vi "Text control 2 v3.0.vi"() -> ()   [LabVIEW 2016]
panel:
  in  "Auto Reset":bool
  in  "Reset":bool
  out "Id min vs time":cluster{"Y data in":dbl[], "X data in":dbl[]}[](graph)
  in  "Start Time":dbl caption="Set Start Time (s)"
  out "Total lines":i32
  out "Line running":i32
  in  "byte count":u32=64
  in  "Serial Settings:Serial End Mode for Reads":u16(ring)=2 items=["None", "LastBit", "TermChar"]
  in  "Timeout (ms)":u32=10000
  in  "Enable Termination\nChar (T)":bool=TRUE
  in  "Termination char\n(0xA = '\\n' = LF)\n(0xD = '\\r' = CR)":u8=13 format="%.0x"
  in  "flow control":u16(ring) items=["None"=0, "XON/XOFF"=1, "RTS/CTS"=2, "DTR/DSR"=4]
  in  "stop bits":u16(ring)=10 items=["1.0"=10, "1.5"=15, "2.0"=20]
  in  "parity":u16(ring) items=["None", "Odd", "Even", "Mark", "Space"]
  in  "data bits":u16=8 min=5 max=8 step=1
  in  "VISA resource name":refnum<visa-resource-name>="COM6"
  in  "baud rate":u32=9600
  out "Serial port output":string
  out "error out":errorcluster
  in  "Units":u16(ring) items=["Seconds", "Minutes", "Hours"]
  out "Elapsed Time":dbl caption="Elapsed Time (s)"
  out "Id max vs time":cluster{"Y data in":dbl[], "X data in":dbl[]}[](graph)
  out "Ig":dbl format="%.2e"
  out "Id":dbl format="%.2e"
  out "Is":dbl format="%.2e"
  out "I vs Vg":cluster{"Y data in":dbl[], "X data in":dbl[]}[](graph)
  in  "Panel Controls 2":T1={"Emergency Stop"=refnum, "TransGraph Max"=1e-05, "Text/Graph (text=false)"=TRUE, "TransGraph Min"=1e-11} {"TransGraph Min" format="%.2e"; "TransGraph Max" format="%.2e"}
  out "Command running:":string="#output s 0 0 0 -0.008 0.008 0.002"
  in  "Standby":T2
  in  "Full Reset":bool
  in  "SMU4":cluster{"on/off":bool, "Voltage":dbl} {"Voltage" min=-100.0 max=100.0 format="%.2f"}
  in  "Source/Drain Range":u8(slide)=6 max=11 scale=0.0..11.0
  in  "Source/Drain\nRange mode":u16(ring) items=["Auto", "Limited", "Fixed"]
  in  "Gate Range":u8(slide)=6 max=11 scale=0.0..11.0
  in  "Gate Range\nmode":u16(ring) items=["Auto", "Limited", "Fixed"]
  in  "Gate":T3={"Gate Start"=0.0, "Gate Stop"=2.0, "Gate Step (linear only)"=1.0, "Gate Compliance"=0.0001, "Gate PComp"=0.0, "Range mode"=0, "Range"=6} {"Range" max=11 scale=0.0..11.0; "Range mode" items=["Auto", "Limited", "Fixed"]; "Gate PComp" format="%^.2e"; "Gate Compliance" format="%^.2e"; "Gate Step (linear only)" format="%^.4e"; "Gate Stop" format="%^.4e"; "Gate Start" format="%^.4e"}
  in  "Drain 2":T4={"Drain Start"=0.0, "Drain Stop"=2.0, "Drain Compliance"=0.0001, "Drain Step"=1.0, "Drain PComp"=0.0, "Range mode"=0, "Range"=6} {"Range" max=11 scale=0.0..11.0; "Range mode" items=["Auto", "Limited", "Fixed"]; "Drain PComp" format="%^.2e"; "Drain Step" format="%^.4e"; "Drain Compliance" format="%^.2e"; "Drain Stop" format="%^.4e"; "Drain Start" format="%^.4e"}
  in  "Timings 2":T5={"integration time"=0, "Short/Long integration time"=0.00064, "hold time (sec)"=0.0, "delay time (sec)"=0.0, "Step Time (0 disables)"=0.0, "sweep method"=0, "Pulse period"=0.005, "Base voltage"=0.0, "Pulse width"=0.0005} {"Pulse width" min=0.0005 max=0.1 step=0.0001 format="%.4f"; "Base voltage" format="%^.4e"; "Pulse period" min=0.005 max=1.0 step=0.0001 format="%.4f"; "sweep method" items=["Continuous", "Pulsed"]; "Step Time (0 disables)" format="%.2f"; "delay time (sec)" format="%.4f"; "hold time (sec)" format="%.4f"; "Short/Long integration time" format="%^.0e"; "integration time" scale=0.0..2.0}
  in  "Panel Controls":T6={"Emergency Stop"=refnum, "TransGraph Max"=1e-05, "Text/Graph (text=false)"=TRUE} {"TransGraph Max" format="%.2e"}
  in  "Interrupt run":bool
  in  "Drain: Compliance":dbl=0.001 format="%.8f"
  in  "Gate: Compliance":dbl=0.001 format="%.8f"
  out "Path":path=path "C:/users/rlp38/09Apr2009LTtesting/test2.txt"
  in  "hold time /s":dbl format="%.2f"
  in  "delay time /s":dbl format="%.2f"
  in  "integration time":u32(slide) max=2 step=1 scale=0.0..2.0
  in  "Integration time (short)":dbl=0.0019 min=8e-05 max=0.0019 step=8e-05 format="%^.0e"
  in  "Integration time (long)":dbl=0.32 min=0.04 max=2.0 step=0.02 format="%.2f"
  in  "Step delay /s":dbl format="%.2f"
  in  "Program":string="#pulsedstressV d 0.03 20 0 0.5 0.0827 5\n#\n#itime s\n#gaterangemode l\n#drainrangemode l\n#pulsed on 0.05 0 0.02\n#transfer d 1 -1 -0.1 -1 -1 0\n#wait-min 1\n#transfer d 1 -1 -0.1 -1 -1 0\n#output d 0 -1 -0.5 0 -1 -0.1\n#transfer d -10 40 1 5 40 35\n#transfer d -10 40 1 5 40 35\n#output d 0 40 20 0 40 1\n#\n#\n#sample 1 0.008 221 6 0.003\n#samplei 400e-6 200 6 0.002 0.1\n#vsu2pulse -10 4\n#\n#stressV 0.016 0.03 2e-4 0.1e-3 11\n#stressI 220e-7 0.08 15\n#transfer s -1 1 0.5 -0.005 0.005 0.005\n#output s 0 0 0 -0.008 0.008 0.002\n"
  # "Serial port settings"
  # "Time"
  # "100 samples is approx 13s with medium integration"
  # "Syntax:\nitime [s|m|l]\ngaterangemode [a|l|f]\ndrainrangemode [a|l|f]\npulsed [on|off] PulsePeriod(sec) PulseBaseVoltage PulseONWidth(sec)\nstandby [on l off]\nwait NumMilliseconds\nwait-min NumMinutes\n# texthere = comment\ntransfer [s|d] VgStart VgStop VgStep VdStart VdStop VdStep\noutput [s|d] VgStart VgStop VgStep VdStart VdStop VdStep\nsample Vg Vd NumSamples Time(s) SampleInterval(s)\nsamplei Idg NumSamples Time(s) SampleInterval(s) VDGcompliance\n# if in doubt use SampleInterval(s) = 0.004\nstressV VG VD IGcompliance IDcompliance Duration(sec)\nstressI IDG VDGcompliance Duration(sec)\nvsu2pulse Bias Duration(s)\npulsedstressV [s|d] VEstop VgON VgOFF Period(s) PulseONwidth(s) Vd\nsample-fpp Vg Vd NumSamples Time\nresample-fpp Vg Vd\ntransfer-fpp [s|d] VgStart VgStop VgStep VdStart VdStop VdStep\noutput-fpp [s|d] VgStart VgStop VgStep VdStart VdStop VdStep\nserial SerialPortCommand"
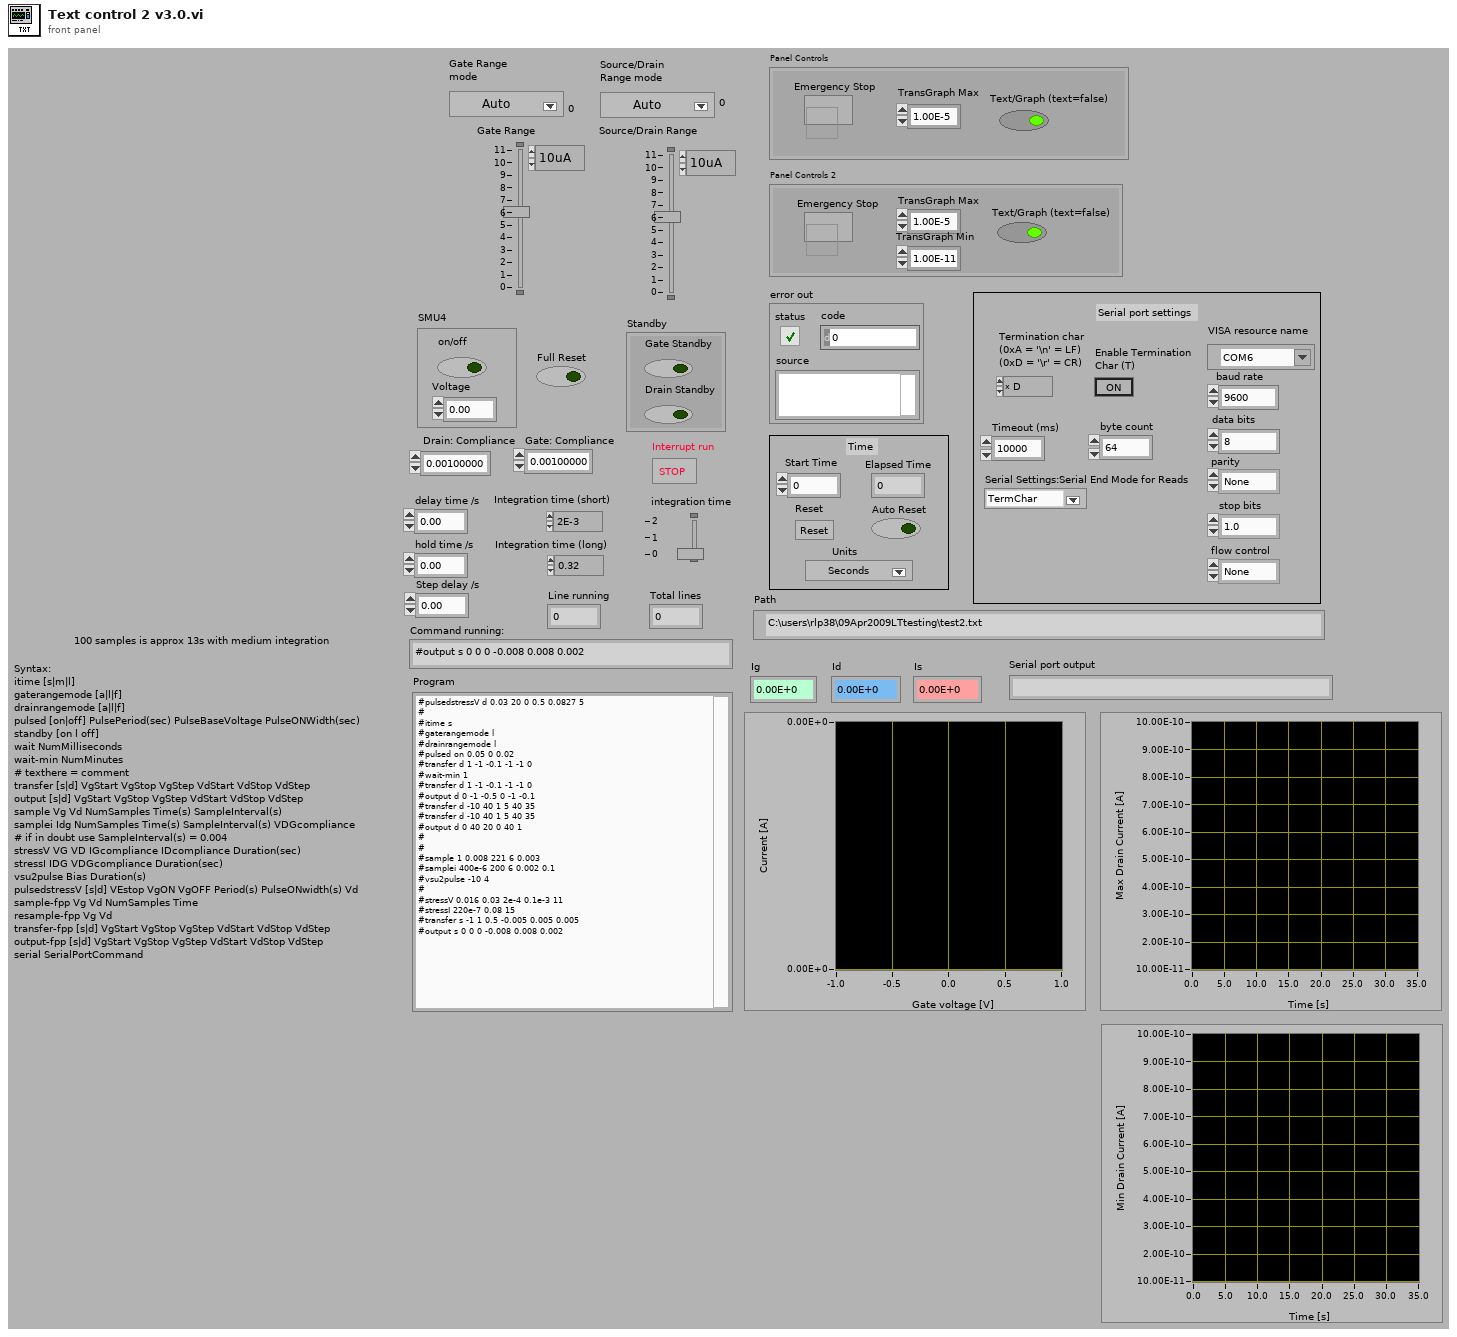
[diagram p1: front panel]
types:
  T1 = cluster{"Emergency Stop":refnum<vi>, "TransGraph Max":dbl, "Text/Graph (text=false)":bool, "TransGraph Min":dbl}
  T2 = cluster{"Gate Standby":bool, "Drain Standby":bool}
  T3 = cluster{"Gate Start":dbl, "Gate Stop":dbl, "Gate Step (linear only)":dbl, "Gate Compliance":dbl, "Gate PComp":dbl, "Range mode":u16, "Range":u8}
  T4 = cluster{"Drain Start":dbl, "Drain Stop":dbl, "Drain Compliance":dbl, "Drain Step":dbl, "Drain PComp":dbl, "Range mode":u16, "Range":u8}
  T5 = cluster{"integration time":u32, "Short/Long integration time":dbl, "hold time (sec)":dbl, "delay time (sec)":dbl, "Step Time (0 disables)":dbl, "sweep method":u16, "Pulse period":dbl, "Base voltage":dbl, "Pulse width":dbl}
  T6 = cluster{"Emergency Stop":refnum<vi>, "TransGraph Max":dbl, "Text/Graph (text=false)":bool}
  T7 = enum16{"open", "replace", "create", "open or create", "replace or create", "replace or create with confirmation"}
  T8 = cluster{"V2 Start":dbl, "V2 Step":dbl, "Number of points":i32}
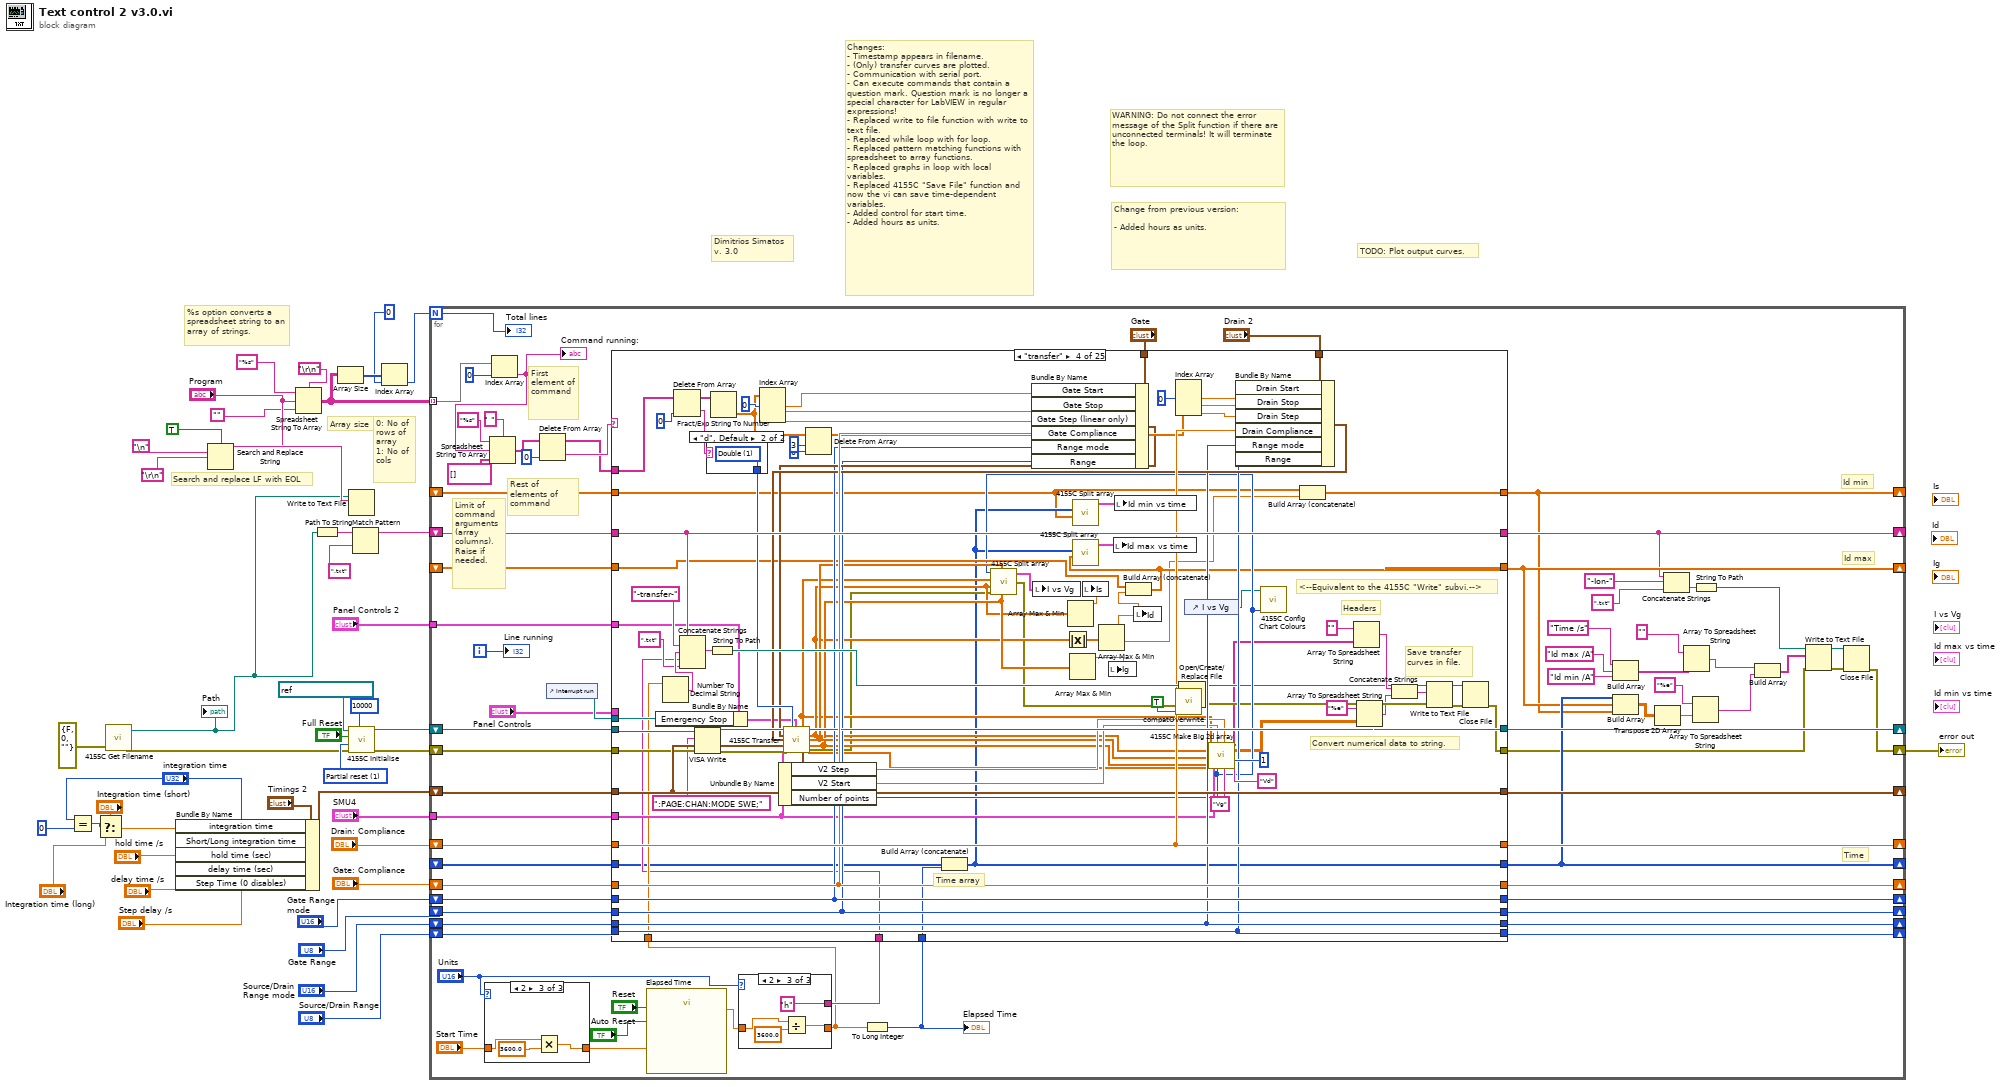
[diagram p0: block diagram]
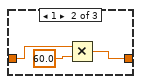
[diagram p3: hidden frame]
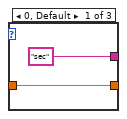
[diagram p4: hidden frame]
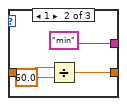
[diagram p5: hidden frame]
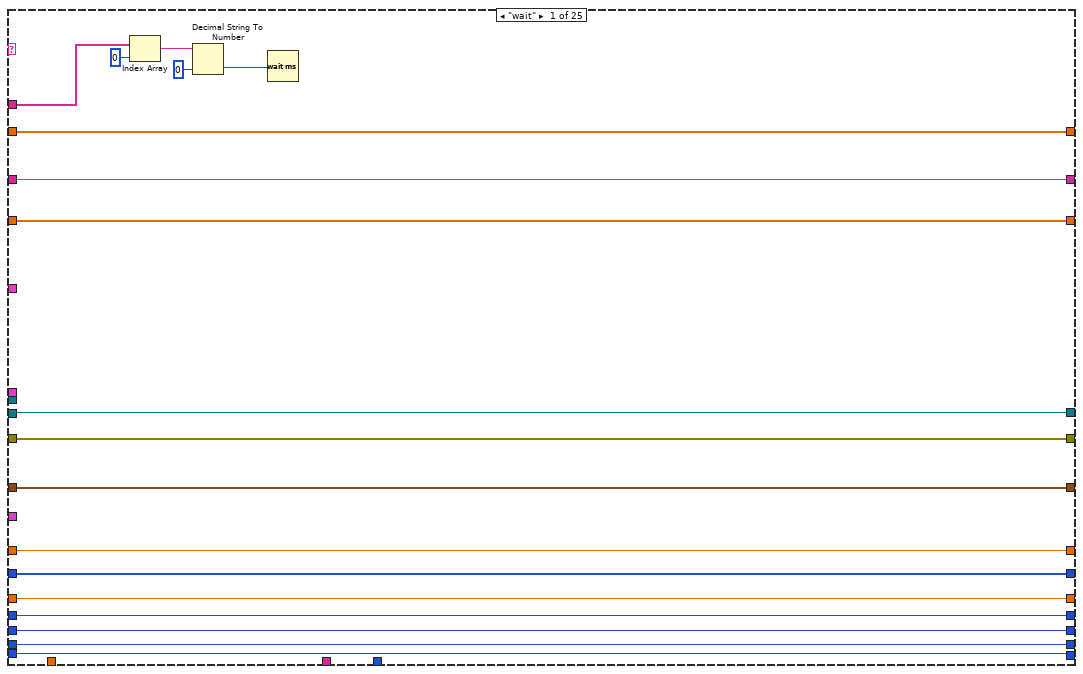
[diagram p6: hidden frame]
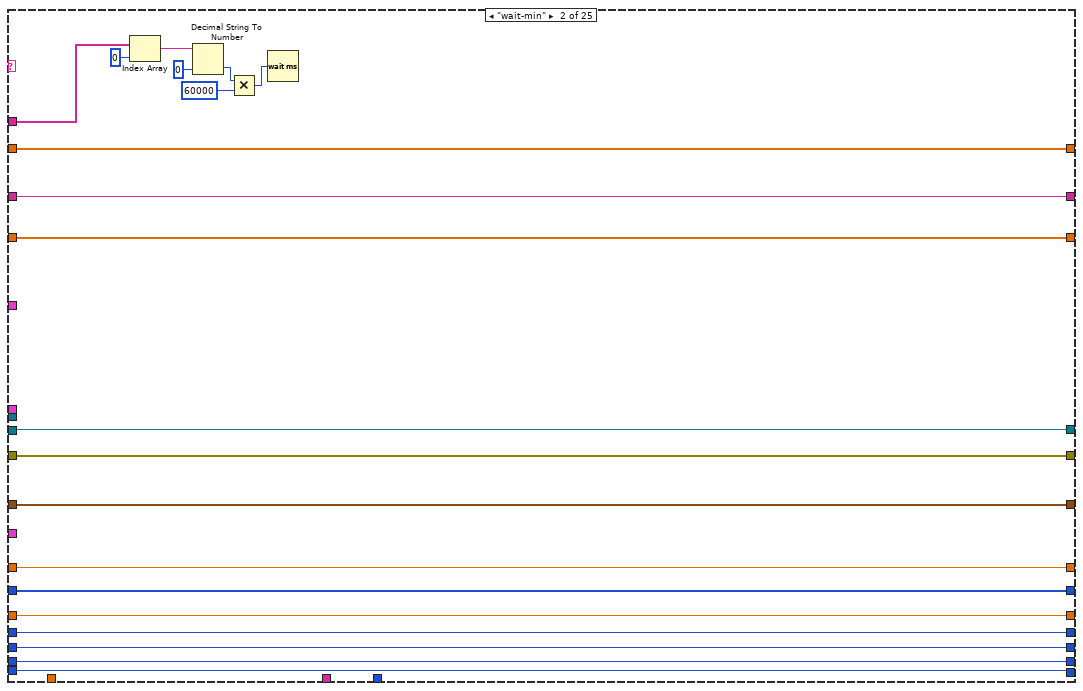
[diagram p7: hidden frame]
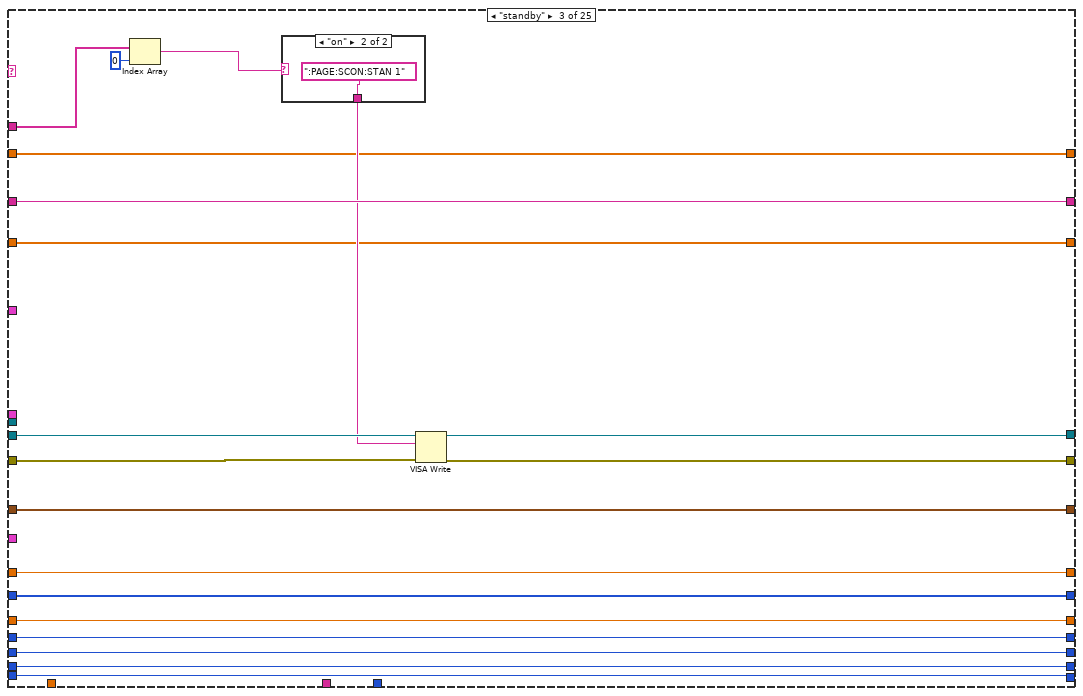
[diagram p8: hidden frame]
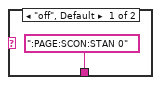
[diagram p9: hidden frame]
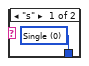
[diagram p10: hidden frame]
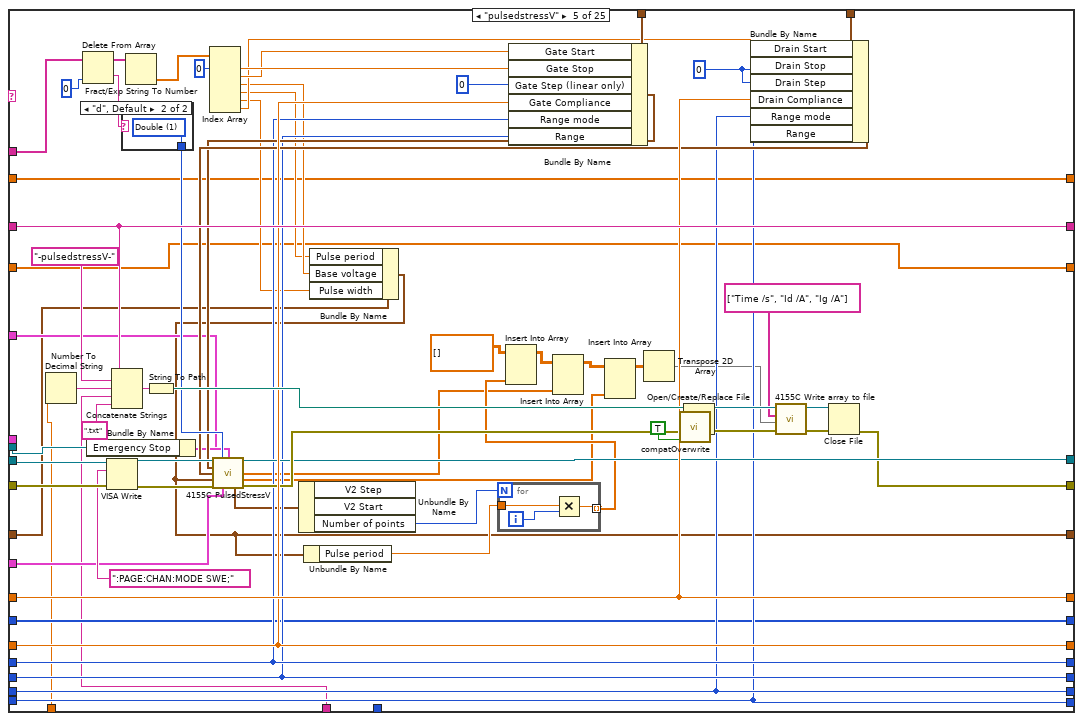
[diagram p11: hidden frame]
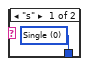
[diagram p12: hidden frame]
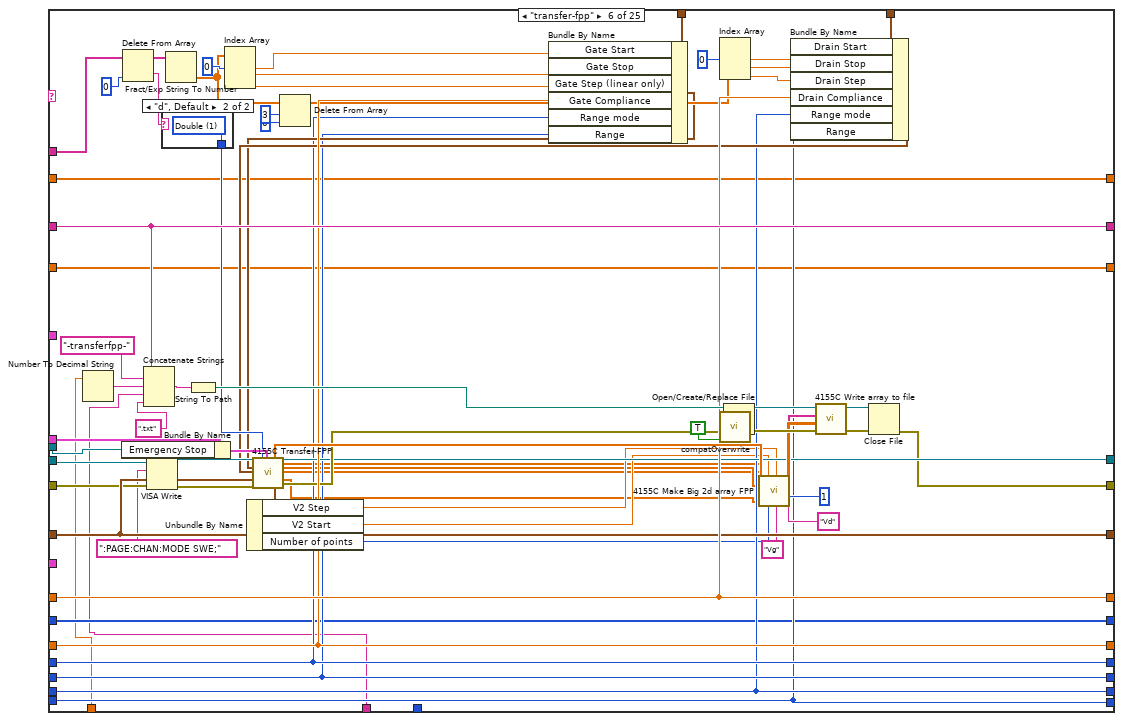
[diagram p13: hidden frame]
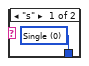
[diagram p14: hidden frame]
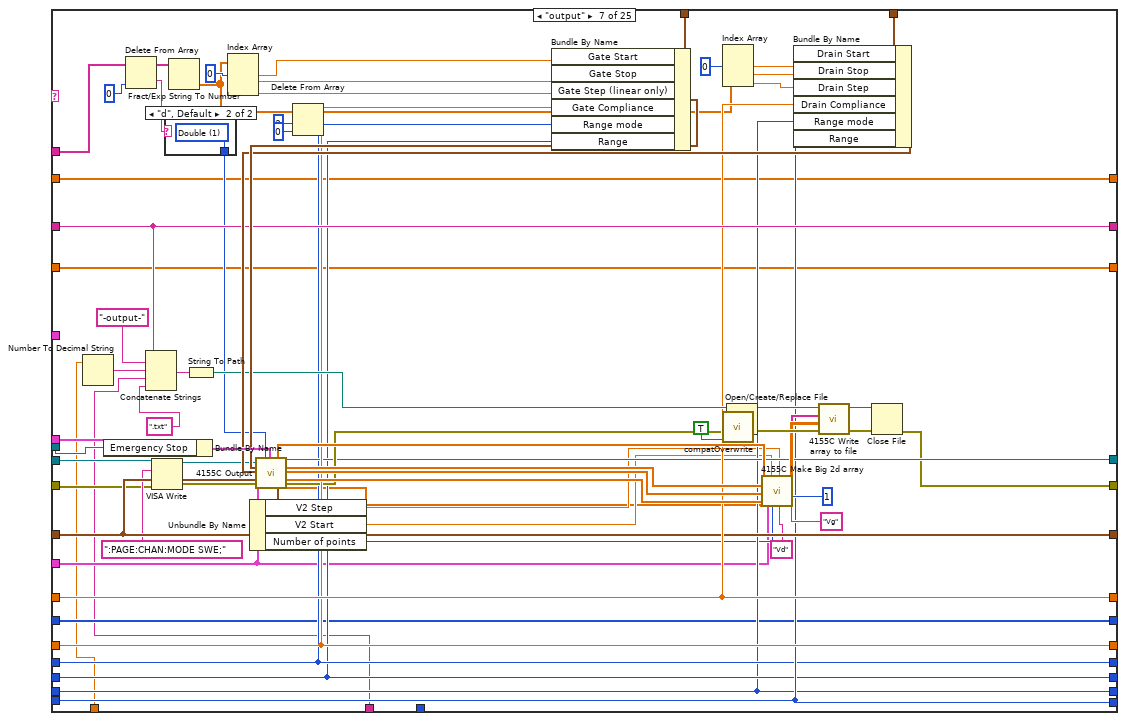
[diagram p15: hidden frame]
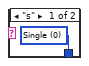
[diagram p16: hidden frame]
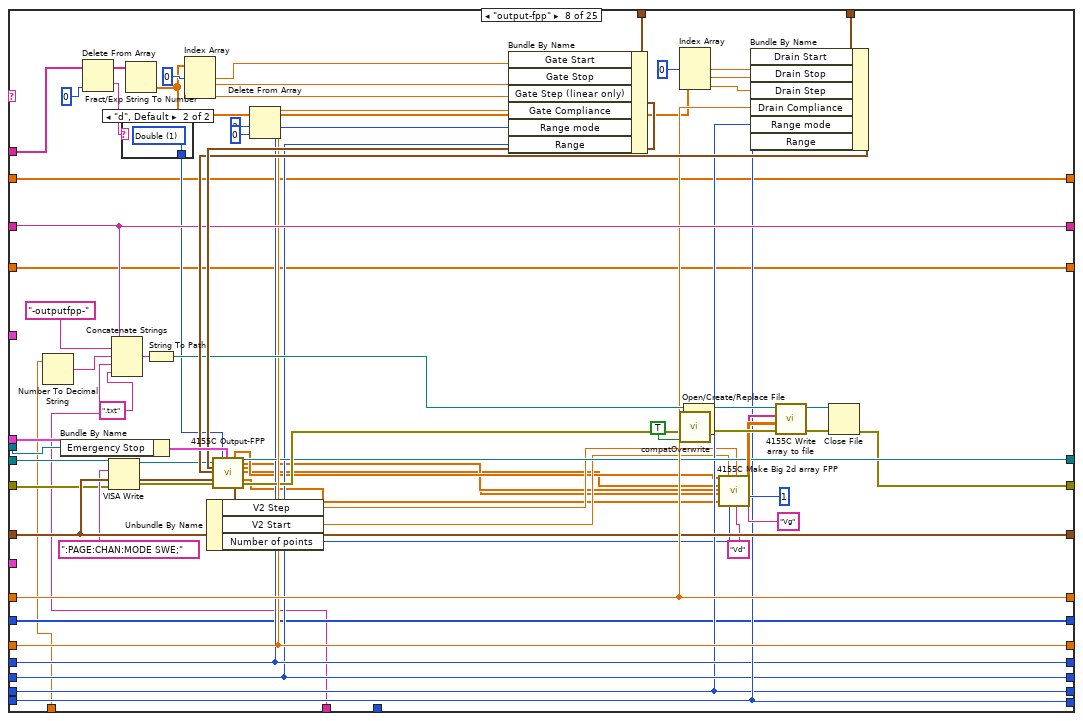
[diagram p17: hidden frame]
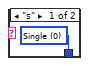
[diagram p18: hidden frame]
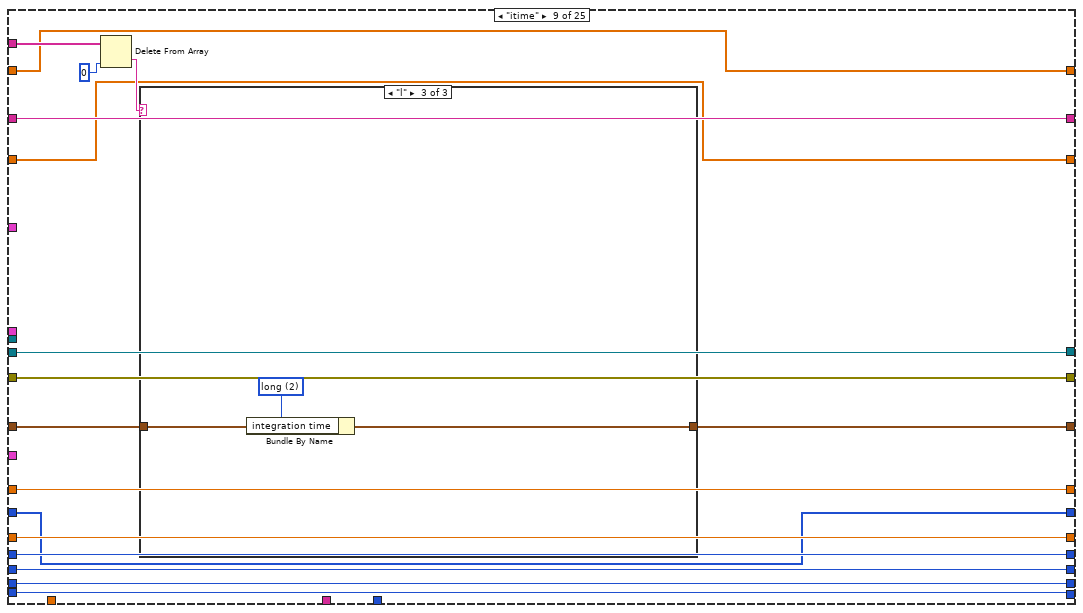
[diagram p19: hidden frame]
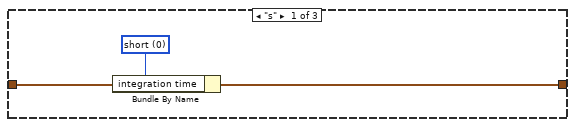
[diagram p20: hidden frame]
diagram:
  w35 = u16 1 items=["Reset All", "Partial reset"] ("Type of reset")
  # "TODO: Plot output curves."
  # "WARNING: Do not connect the error message of the Split function if there are unconnected terminals! It will terminate the loop."
  # "Array size"
  # "%s option converts a spreadsheet string to an array of strings."
  # "0: No of rows of array\n1: No of cols"
  # "Change from previous version:\n\n- Added hours as units."
  # "Dimitrios Simatos\nv. 3.0"
  # "Changes:\n- Timestamp appears in filename.\n- (Only) transfer curves are plotted.\n- Communication with serial port.\n- Can execute commands that contain a question mark. Question mark is no longer a special character for LabVIEW in regular expressions!\n- Replaced write to file function with write to text file.\n- Replaced while loop with for loop.\n- Replaced pattern matching functions with spreadsheet to array functions.\n- Replaced graphs in loop with local variables.\n- Replaced 4155C \"Save File\" function and now the vi can save time-dependent variables.\n- Added control for start time.\n- Added hours as units."
  # "Search and replace LF with EOL"
  n1 = Equal?(x="integration time", y=u32 0) -> (x = y?=w39:bool)
  n2 = Select(t="Integration time (short)", s=w39, f="Integration time (long)") -> (s? t:f=w43:dbl)
  n3 = call "4155C Get Filename.vi"("error in (no error)"=errorcluster {"status"=FALSE, "code"=0, "source"=""}) -> ("error out"=w30:errorcluster, "path"=w2:path)  [unwired: 2 in, 1 out]
  "Path" <- w2
  n4 = Bundle By Name(cluster="Timings 2", "integration time"="integration time", "Short/Long integration time"=w43, "hold time (sec)"="hold time /s", "delay time (sec)"="delay time /s", "Step Time (0 disables)"="Step delay /s") -> (w27:T5)
  n5 = Search and Replace String(replace all?=TRUE ("replace all? (F)"), input string="Program", search string="\n", replace string="\r\n") -> (result string=w17:string)  [unwired: 4 in, 3 out]
  n6 = Spreadsheet String To Array(delimiter (Tab)="\r\n", format string="%s", spreadsheet string="Program", array type (2D Dbl)="") -> (array=w8:string[][])
  n7 = Path To String(path=w2) -> (string=w5:string)
  n8 = Array Size(array=w8) -> (size(s)=w12:i32[])
  n9 = Write to Text File(file (use dialog)=w2, text=w17) -> ()  [unwired: 2 in, 3 out]
  n10 = call "4155C Initialise.vi"("VISA resource name in"=refnum<visa-resource-name> "GPIB0::14::INSTR", "Reset"="Full Reset", "Type of reset"=w35, "error in (no error)"=w30, "VISA Timeout Value"=u32 10000) -> ("VISA Resource Name out"=w29:refnum<visa-resource-name>, "error out"=w28:errorcluster)
  n11 = Match Pattern(string=w5, regular expression=".txt") -> (before substring=w3:string)  [unwired: 1 in, 3 out]
  n12 = Index Array(array=w12, index=0) -> (element=w10:i32)
  n13 = for {
    N: w10 -> [w81]
    tunnel: "SMU4" -> [w93]
    shift-left: "Source/Drain Range" -> [w98]
    shift-right: [w94] -> _
    shift-left: "Source/Drain\nRange mode" -> [w99]
    shift-right: [w95] -> _
    shift-left: "Gate Range" -> [w100]
    shift-right: [w96] -> _
    shift-left: "Gate Range\nmode" -> [w101]
    shift-right: [w97] -> _
    shift-left: "Gate: Compliance" -> [w110]
    shift-right: [w106] -> _
    shift-left: "Drain: Compliance" -> [w111]
    shift-right: [w107] -> _
    shift-left: w27 -> [w112]
    shift-right: [w108] -> _
    shift-left: w28 -> [w113]
    shift-right: [w50] -> w1
    shift-left: w29 -> [w114]
    shift-right: [w109] -> _
    shift-left: w3 -> [w115]
    shift-right: [w54] -> _
    tunnel: "Panel Controls 2" -> [w92]
    shift-right: [w57] -> _
    shift-left: _ -> [w91]
    shift-right: [w58] -> _
    shift-left: _ -> [w87]
    tunnel: w8 -> [w84] mode=indexing
    shift-right: [w48] -> _
    shift-left: _ -> [w49]
    i -> [w82]
    # "Time"
    # "Rest of elements of command"
    # "Id min"
    # "Id max"
    # "Limit of command arguments (array columns). Raise if needed."
    # "First element of command"
    n14 = case shown="2" "Units" {
      tunnel: "Start Time" -> [w116 w119 w122]
      tunnel: [w116 w118 w121] -> w46
      frame 0, Default {
      }
      frame 1 {
        n15 = Multiply(x=w119, y=60.0) -> (x*y=w118:dbl)
      }
      frame 2 {
        n16 = Multiply(x=w122, y=3600.0) -> (x*y=w121:dbl)
      }
    }
    n17 = Index Array(array=w84, index=0 ("line index")) -> (element=w77:string)
    "Command running:" <- w77
    n18 = Spreadsheet String To Array(delimiter (Tab)=" ", format string="%s", spreadsheet string=w77, array type (2D Dbl)=string[] []) -> (array=w74:string[])
    n19 = Delete From Array(array=w74, index=0) -> (deleted portion=w75:string, array with subset deleted=w73:string[])  [unwired: 1 in]
    n20 = control-ref of="Interrupt run"() -> (w105:refnum<vi>)
    n21 = call "Elapsed Time"("Reset"="Reset", "Auto Reset"="Auto Reset", "Set Start Time (s)"=w46) -> ("Elapsed Time (s)"=w88:dbl)  [unwired: 9 in, 7 out]
    n22 = case shown="2" "Units" {
      tunnel: ["sec" "min" "h"] -> w89
      tunnel: [w123 w127 w130] -> w86
      tunnel: w88 -> [w123 w126 w131]
      frame 0, Default {
      }
      frame 1 {
        n23 = Divide(x=w126, y=60.0) -> (x/y=w127:dbl)
      }
      frame 2 {
        n24 = Divide(x=w131, y=3600.0) -> (x/y=w130:dbl)
      }
    }
    n25 = To Long Integer(number=w86) -> (32bit integer=w85:i32)
    "Elapsed Time" <- w85
    n26 = case shown="\"transfer\"" w75 {
      tunnel: w73 -> [w150 w170 w189 w270 w335 w405 w473 w549 w588 w615 w643 w669 w691 w706 _ _ w813 w875 _ w942 w987 w1030 w1101 w1164 w1172]
      tunnel: w115 -> [w145 w166 w187 w277 w342 w413 w481 w557 w577 w604 w635 w662 w685 w699 w719 w762 w791 w857 w889 w929 w974 w1018 w1095 w1160 w1174]
      tunnel: w114 -> [w144 w165 w178 w248 w326 w382 w449 w525 w578 w605 w636 w663 w686 w700 w724 w764 w819 w881 w893 w948 w993 w1036 w1107 w1118 w1178]
      tunnel: w113 -> [w143 w164 w177 w247 w325 w381 w446 w522 w579 w606 w637 w664 w687 w701 w723 w735 w818 w880 w892 w947 w992 w1035 w1106 w1117 w1177]
      tunnel: w112 -> [w142 w163 w186 w273 w301 w409 w477 w553 w587 w614 w634 w661 w684 w698 w722 w759 w782 w849 w898 w922 w967 w1011 w1094 w1159 w1179]
      tunnel: w111 -> [w141 w162 w185 w275 w340 w411 w479 w555 w586 w613 w642 w668 w690 w705 w721 w744 w817 w879 w901 w946 w991 w1034 w1105 w1168 w1180]
      tunnel: w110 -> [w140 w161 w184 w274 w339 w410 w478 w554 w585 w612 w641 w667 w689 w704 w720 w745 w792 w858 w900 w930 w975 w1019 w1096 w1161 w1182]
      tunnel: [w144 w165 w176 w272 w337 w407 w475 w551 w578 w605 w636 w663 w686 w700 w724 w764 w783 w831 w891 w923 w968 w1012 w1047 w1120 w1178] -> w109
      tunnel: [w143 w164 w175 w271 w336 w406 w474 w550 w579 w606 w637 w664 w687 w701 w723 w734 w793 w832 w890 w931 w976 w1020 w1046 w1119 w1176] -> w51
      tunnel: [w142 w163 w186 w273 w297 w409 w477 w553 w580 w607 w634 w661 w684 w698 w722 w759 w782 w849 w898 w922 w967 w1011 w1094 w1159 w1179] -> w108
      tunnel: [w141 w162 w185 w275 w340 w411 w479 w555 w586 w613 w642 w668 w690 w705 w721 w744 w817 w879 w901 w946 w991 w1034 w1105 w1168 w1180] -> w107
      tunnel: [w140 w161 w184 w274 w339 w410 w478 w554 w585 w612 w641 w667 w689 w704 w720 w745 w792 w858 w900 w930 w975 w1019 w1096 w1161 w1182] -> w106
      tunnel: [w145 w166 w187 w277 w342 w413 w481 w557 w577 w604 w635 w662 w685 w699 w719 w762 w791 w857 w889 w929 w974 w1018 w1095 w1160 w1174] -> w54
      tunnel: w105 -> [_ _ _ w280 w346 w418 w489 w561 _ _ _ _ _ _ _ _ w788 w854 _ w928 w973 w1017 w1067 w1136 _]
      tunnel: "Gate" -> [_ _ _ w257 w329 w392 w460 w536 _ _ _ _ _ _ _ _ _ _ _ _ _ _ _ _ _]
      tunnel: "Drain 2" -> [_ _ _ w256 w328 w391 w459 w535 _ _ _ _ _ _ _ _ _ _ _ _ _ _ _ _ _]
      tunnel: "Panel Controls" -> [_ _ _ _ _ w390 w458 w534 _ _ _ _ _ _ _ _ _ _ _ _ _ _ _ _ _]
      tunnel: w101 -> [w139 w160 w183 w241 w319 w375 w444 w520 w584 w611 _ w660 w683 w697 w718 w746 w778 w845 w894 w918 w963 w1007 w1090 w1155 w1183]
      tunnel: w100 -> [w138 w159 w182 w240 w318 w374 w443 w519 w583 w610 w640 _ w674 w703 w717 w747 w779 w846 w895 w919 w964 w1008 w1091 w1156 w1184]
      tunnel: w99 -> [w137 w158 w181 w239 w317 w373 w442 w518 w582 w609 w639 w666 w688 _ w716 w748 w780 w847 w896 w920 w965 w1009 w1092 w1157 w1185]
      tunnel: w98 -> [w136 w157 w180 w238 w316 w372 w445 w521 w581 w608 w638 w665 _ w702 w715 w749 w781 w848 w897 w921 w966 w1010 w1093 w1158 w1186]
      tunnel: [w139 w160 w183 w241 w319 w375 w444 w520 w584 w611 w633 w660 w683 w697 w718 w746 w778 w845 w894 w918 w963 w1007 w1090 w1155 w1183] -> w97
      tunnel: [w138 w159 w182 w240 w318 w374 w443 w519 w583 w610 w640 w652 w674 w703 w717 w747 w779 w846 w895 w919 w964 w1008 w1091 w1156 w1184] -> w96
      tunnel: [w137 w158 w181 w239 w317 w373 w442 w518 w582 w609 w639 w666 w688 w696 w716 w748 w780 w847 w896 w920 w965 w1009 w1092 w1157 w1185] -> w95
      tunnel: [w136 w157 w180 w238 w316 w372 w445 w521 w581 w608 w638 w665 w675 w702 w715 w749 w781 w848 w897 w921 w966 w1010 w1093 w1158 w1186] -> w94
      tunnel: w93 -> [_ _ _ w233 w313 _ w437 _ _ _ _ _ _ _ _ _ _ _ _ _ _ _ _ _ _]
      tunnel: w92 -> [_ _ _ w231 w312 _ _ _ _ _ _ _ _ _ _ _ _ _ _ _ _ _ _ _ _]
      tunnel: [w135 w153 w173 w199 w289 w362 w434 w507 w576 w602 w632 w651 w673 w695 w714 w730 w770 w829 w888 w907 w956 w1001 w1044 w1113 w1175] -> w57
      tunnel: w91 -> [w135 w153 w173 w222 w289 w362 w434 w507 w576 w602 w632 w651 w673 w695 w714 w730 w770 w829 w888 w907 w956 w1001 w1044 w1113 w1175]
      tunnel: w86 -> [_ _ _ w218 w286 w360 w431 w504 _ _ _ _ _ _ _ w728 w768 w826 _ w904 w953 w998 w1041 w1109 _]
      tunnel: w89 -> [_ _ _ w215 w285 w358 w430 w503 _ _ _ _ _ _ _ w726 w766 w825 _ w903 w952 w997 w1040 w1110 _]
      tunnel: w85 -> [_ _ _ w200 _ _ _ _ _ _ _ _ _ _ _ _ _ _ _ _ _ _ _ _ _]
      tunnel: [w134 w152 w172 w195 w288 w361 w433 w506 w575 w601 w631 w650 w672 w694 w713 w729 w769 w828 w887 w906 w955 w1000 w1043 w1112 w1181] -> w58
      tunnel: w87 -> [w134 w152 w172 w214 w288 w361 w433 w506 w575 w601 w631 w650 w672 w694 w713 w729 w769 w828 w887 w906 w955 w1000 w1043 w1112 w1181]
      tunnel: [w133 w151 w171 w193 w284 w357 w429 w502 w574 w600 w630 w649 w671 w693 w712 w725 w765 w824 w886 w902 w951 w996 w1039 w1108 w1169] -> w48
      tunnel: w49 -> [w133 w151 w171 w192 w284 w357 w429 w502 w574 w600 w630 w649 w671 w693 w712 w725 w765 w824 w886 w902 w951 w996 w1039 w1108 w1169]
      frame "wait" {
        n27 = Index Array(array=w150, index=0 ("Index")) -> (element=w148:string)
        n28 = Decimal String To Number(string=w148, default (0L)=u32 0) -> (number=w147:u32)  [unwired: 1 in, 1 out]
        n29 = Wait (ms)(milliseconds to wait=w147) -> ()  [unwired: 1 out]
      }
      frame "wait-min" {
        n30 = Index Array(array=w170, index=0 ("Index")) -> (element=w168:string)
        n31 = Decimal String To Number(string=w168, default (0L)=u32 0) -> (number=w156:u32)  [unwired: 1 in, 1 out]
        n32 = Multiply(x=w156, y=u32 60000) -> (x*y=w155:u32)
        n33 = Wait (ms)(milliseconds to wait=w155) -> ()  [unwired: 1 out]
      }
      frame "standby" {
        n34 = Index Array(array=w189, index=0 ("Index")) -> (element=w179:string)
        n35 = case shown="\"on\"" w179 {
          tunnel: [":PAGE:SCON:STAN 0" ":PAGE:SCON:STAN 1"] -> w174
          frame "off", Default {
          }
          frame "on" {
          }
        }
        n36 = VISA Write(VISA resource name=w178, write buffer=w174, error in (no error)=w177) -> (VISA resource name out=w176:refnum<visa-resource-name>, error out=w175:errorcluster)  [unwired: 1 out]
      }
      frame "transfer" {
        # "<--Equivalent to the 4155C \"Write\" subvi.-->"
        # "Headers"
        # "Convert numerical data to string."
        # "Save transfer curves in file."
        # "Time array"
        n37 = Bundle By Name(cluster=w231, "Emergency Stop"=w280) -> (w232:T1)
        n38 = Number To Decimal String(number=w218) -> (decimal integer string=w217:string)  [unwired: 1 in]
        n39 = Delete From Array(array=w270, index=0 ("Index")) -> (deleted portion=w268:string, array with subset deleted=w267:string[])  [unwired: 1 in]
        n40 = Concatenate Strings(w277, "-transfer-" ("Prefix"), w217, w215, ".txt" ("Suffix")) -> (w279:string)
        n41 = VISA Write(VISA resource name=w248, write buffer=":PAGE:CHAN:MODE SWE;" ("write buffer (\"\")"), error in (no error)=w247) -> (VISA resource name out=w245:refnum<visa-resource-name>, error out=w246:errorcluster)  [unwired: 1 out]
        n42 = case shown="\"d\", Default" w268 {
          tunnel: [w282 w283] -> w266
          frame "s" {
            w282 = u16 0 items=["Single", "Double"] ("sweep mode")
          }
          frame "d", Default {
            w283 = u16 1 items=["Single", "Double"] ("sweep mode")
          }
        }
        n43 = String To Path(string=w279) -> (path=w276:path)
        n44 = Fract/Exp String To Number(string=w267) -> (number=w252:dbl[])  [unwired: 3 in, 1 out]
        n45 = Index Array(array=w252, index #1=0 ("Index")) -> (element #1=w265:dbl, element #2=w264:dbl, element #3=w263:dbl)  [unwired: 2 in]
        n46 = Delete From Array(array=w252, length=3 ("Length"), index=0 ("Index")) -> (array with subset deleted=w250:dbl[])  [unwired: 1 out]
        n47 = Build Array (concatenate)(w214, w200) -> (w195:i32[])
        n48 = Bundle By Name(cluster=w257, "Gate Start"=w265, "Gate Stop"=w264, "Gate Step (linear only)"=w263, "Gate Compliance"=w274, "Range mode"=w241, "Range"=w240) -> (w242:T3)
        n49 = call "4155C Split array.vi"("X data in"=w195, "Y1 data in"=w192) -> ("Array of clusters"=w196:cluster{"Y data in":dbl[], "X data in":dbl[]}[])  [unwired: 5 in, 1 out]
        n50 = local write "Id min vs time"(w196) -> ()
        n51 = Index Array(array=w250, index #1=0 ("Index")) -> (element #1=w260:dbl, element #2=w259:dbl, element #3=w258:dbl)  [unwired: 2 in]
        n52 = call <vilib>:"compatOverwrite.vi"("overwrite (F)"=TRUE) -> ("overwrite?"=w230:T7)
        n53 = control-ref of="I vs Vg"() -> (w219:refnum<vi>)
        n54 = Bundle By Name(cluster=w256, "Drain Start"=w260, "Drain Stop"=w259, "Drain Step"=w258, "Drain Compliance"=w275, "Range mode"=w239, "Range"=w238) -> (w243:T4)
        n55 = call "4155C Transfer.vi"("VISA resource name in"=w245, "Gate"=w242, "Drain"=w243, "Timings"=w273, "error in (no error)"=w246, "SMU4"=w233, "sweep mode"=w266, "Panel Controls"=w232) -> ("VG"=w223:dbl[], "Outparams"=w237:T8, "VISA Resource Name out"=w272:refnum<visa-resource-name>, "IS"=w224:dbl[], "ID"=w229:dbl[], "IG"=w225:dbl[], "error out"=w210:errorcluster, "SMU4"=w234:dbl[])  [unwired: 12 in]
        n56 = Unbundle By Name(w237) -> ("V2 Step"=w236:dbl, "V2 Start"=w235:dbl, "Number of points"=w220:i32)
        n57 = call "4155C Split array.vi"("Number of VAR2 steps"=w220, "Y2 data in"=w229, "X data in"=w223, "Y1 data in"=w224, "Y3 data in"=w225, "error in (no error)"=w210) -> ("Array of clusters"=w213:cluster{"Y data in":dbl[], "X data in":dbl[]}[], "error out"=w211:errorcluster)  [unwired: 1 in]
        n58 = local write "I vs Vg"(w213) -> ()
        n59 = Absolute Value(x=w224) -> (abs(x)=w228:dbl[])
        n60 = Array Max & Min(array=w224) -> (max value=w226:dbl)  [unwired: 3 out]
        n61 = Array Max & Min(array=w225) -> (max value=w227:dbl)  [unwired: 3 out]
        n62 = local write "Is"(w226) -> ()
        n63 = Array Max & Min(array=w228) -> (max value=w221:dbl, min value=w194:dbl)  [unwired: 2 out]
        n64 = local write "Ig"(w227) -> ()
        n65 = Build Array (concatenate)(w222, w221) -> (w199:dbl[])
        n66 = call "4155C Split array.vi"("X data in"=w195, "Y1 data in"=w199) -> ("Array of clusters"=w212:cluster{"Y data in":dbl[], "X data in":dbl[]}[])  [unwired: 5 in, 1 out]
        n67 = local write "Id max vs time"(w212) -> ()
        n68 = local write "Id"(w221) -> ()
        n69 = Open/Create/Replace File(file path (use dialog)=w276, error in=w211, operation (0:open)=w230) -> (refnum out=w198:refnum<file>, error out=w207:errorcluster)  [unwired: 3 in, 1 out]
        n70 = call "4155C Make Big 2d array.vi"("1D Var1"=w223, "1d IS"=w224, "1d ID"=w229, "1d IG"=w225, "1d SMU4"=w234, "SMU4"=w233, "VAR2 START"=w235, "Number of VAR2 steps"=w220, "VAR2 STEP"=w236, "VAR1 Name"="Vg", "Decimal places in header"=i8 1, "VAR2 Name"="Vd") -> ("Header array"=w197:string[], "Data array"=w204:dbl[][])  [unwired: 14 in]
        n71 = call "4155C Config Chart Colours.vi"("Numeric"=w220, "XY Graph 2"=w219) -> ()  [unwired: 6 in]
        n72 = Build Array (concatenate)(w192, w194) -> (w193:dbl[])
        n73 = Array To Spreadsheet String(array=w197, 3:"" ("format string")) -> (spreadsheet string=w203:string)  [unwired: 1 in]
        n74 = Array To Spreadsheet String(array=w204, 3:"%e" ("format string")) -> (spreadsheet string=w206:string)  [unwired: 1 in]
        n75 = Concatenate Strings(w203, w206) -> (w205:string)
        n76 = Write to Text File(file (use dialog)=w198, text=w205, error in=w207) -> (refnum out=w209:refnum<file>, error out=w208:errorcluster)  [unwired: 1 in, 1 out]
        n77 = Close File(refnum=w209, error in=w208) -> (error out=w271:errorcluster)  [unwired: 1 out]
      }
      frame "pulsedstressV" {
        w295 = 0
        n78 = Number To Decimal String(number=w286) -> (decimal integer string=w343:string)  [unwired: 1 in]
        n79 = Delete From Array(array=w335, index=0 ("Index")) -> (deleted portion=w333:string, array with subset deleted=w332:string[])  [unwired: 1 in]
        n80 = Bundle By Name(cluster=w312, "Emergency Stop"=w346) -> (w314:T1)
        n81 = VISA Write(VISA resource name=w326, write buffer=":PAGE:CHAN:MODE SWE;" ("write buffer (\"\")"), error in (no error)=w325) -> (VISA resource name out=w323:refnum<visa-resource-name>, error out=w324:errorcluster)  [unwired: 1 out]
        n82 = Concatenate Strings(w342, "-pulsedstressV-" ("Substring"), w343, w285, ".txt" ("Substring")) -> (w345:string)
        n83 = case shown="\"d\", Default" w333 {
          tunnel: [w355 w356] -> w331
          frame "s" {
            w355 = u16 0 items=["Single", "Double"] ("sweep mode")
          }
          frame "d", Default {
            w356 = u16 1 items=["Single", "Double"] ("sweep mode")
          }
        }
        n84 = Fract/Exp String To Number(string=w332) -> (number=w327:dbl[])  [unwired: 3 in, 1 out]
        n85 = String To Path(string=w345) -> (path=w341:path)
        n86 = Index Array(array=w327, index #1=0 ("Index")) -> (element #1=w304:dbl, element #2=w303:dbl, element #3=w300:dbl, element #4=w299:dbl, element #5=w298:dbl, element #6=w302:dbl)  [unwired: 5 in]
        n87 = Bundle By Name(cluster=w301, "Pulse period"=w299, "Base voltage"=w300, "Pulse width"=w298) -> (w297:T5)
        n88 = Unbundle By Name(w297) -> ("Pulse period"=w305:dbl)
        n89 = Bundle By Name(cluster=w329, "Gate Start"=w303, "Gate Stop"=w304, "Gate Step (linear only)"=0, "Gate Compliance"=w339, "Range mode"=w319, "Range"=w318) -> (w320:T3)
        n90 = call <vilib>:"compatOverwrite.vi"("overwrite (F)"=TRUE) -> ("overwrite?"=w290:T7)
        n91 = Bundle By Name(cluster=w328, "Drain Start"=w302, "Drain Stop"=w295, "Drain Step"=w295, "Drain Compliance"=w340, "Range mode"=w317, "Range"=w316) -> (w321:T4)
        n92 = call "4155C PulsedStressV.vi"("VISA resource name in"=w323, "sweep mode"=w331, "Panel Controls"=w314, "Gate"=w320, "Drain"=w321, "Timings"=w297, "error in (no error)"=w324, "SMU4"=w313) -> ("VISA Resource Name out"=w337:refnum<visa-resource-name>, "ID"=w293:dbl[], "IG"=w291:dbl[], "Outparams"=w315:T8, "error out"=w338:errorcluster)  [unwired: 3 in]
        n93 = Unbundle By Name(w315) -> ("Number of points"=w292:i32)  [unwired: 2 out]
        n94 = for {
          N: w292 -> [_]
          tunnel: [w352] -> w294 mode=indexing
          tunnel: w305 -> [w354]
          i -> [w353]
          n95 = Multiply(x=w354, y=w353) -> (x*y=w352:dbl)
        }
        n96 = Insert Into Array(array=dbl[][] [] ("Input Array"), new element=w294) -> (w306:dbl[][])  [unwired: 2 in]
        n97 = Insert Into Array(array=w306, new element=w293) -> (w311:dbl[][])  [unwired: 2 in]
        n98 = Insert Into Array(array=w311, new element=w291) -> (w310:dbl[][])  [unwired: 2 in]
        n99 = Transpose 2D Array(2D array=w310) -> (transposed array=w309:dbl[][])
        n100 = Open/Create/Replace File(file path (use dialog)=w341, error in=w338, operation (0:open)=w290) -> (refnum out=w349:refnum<file>, error out=w350:errorcluster)  [unwired: 3 in, 1 out]
        n101 = call "4155C Write array to file.vi"("Byte Stream File Refnum"=w349, "Header"=string[] ["Time /s", "Id /A", "Ig /A"], "Data Array"=w309, "error in (no error)"=w350) -> ("dup refnum"=w347:refnum<file>, "error out"=w348:errorcluster)  [unwired: 1 in]
        n102 = Close File(refnum=w347, error in=w348) -> (error out=w336:errorcluster)  [unwired: 1 out]
      }
      frame "transfer-fpp" {
        n103 = Number To Decimal String(number=w360) -> (decimal integer string=w414:string)  [unwired: 1 in]
        n104 = Bundle By Name(cluster=w390, "Emergency Stop"=w418) -> (w426:T6)
        n105 = Delete From Array(array=w405, index=0 ("Index")) -> (deleted portion=w403:string, array with subset deleted=w402:string[])  [unwired: 1 in]
        n106 = Concatenate Strings(w413, "-transferfpp-" ("Substring"), w414, w358, ".txt" ("Substring")) -> (w416:string)
        n107 = VISA Write(VISA resource name=w382, write buffer=":PAGE:CHAN:MODE SWE;" ("write buffer (\"\")"), error in (no error)=w381) -> (VISA resource name out=w379:refnum<visa-resource-name>, error out=w380:errorcluster)  [unwired: 1 out]
        n108 = case shown="\"d\", Default" w403 {
          tunnel: [w427 w428] -> w401
          frame "s" {
            w427 = u16 0 items=["Single", "Double"] ("sweep mode")
          }
          frame "d", Default {
            w428 = u16 1 items=["Single", "Double"] ("sweep mode")
          }
        }
        n109 = Fract/Exp String To Number(string=w402) -> (number=w386:dbl[])  [unwired: 3 in, 1 out]
        n110 = String To Path(string=w416) -> (path=w412:path)
        n111 = Index Array(array=w386, index #1=0 ("Index")) -> (element #1=w400:dbl, element #2=w399:dbl, element #3=w398:dbl)  [unwired: 2 in]
        n112 = Delete From Array(array=w386, length=3 ("Length"), index=0 ("Index")) -> (array with subset deleted=w384:dbl[])  [unwired: 1 out]
        n113 = Bundle By Name(cluster=w392, "Gate Start"=w400, "Gate Stop"=w399, "Gate Step (linear only)"=w398, "Gate Compliance"=w410, "Range mode"=w375, "Range"=w374) -> (w376:T3)
        n114 = Index Array(array=w384, index #1=0 ("Index")) -> (element #1=w395:dbl, element #2=w394:dbl, element #3=w393:dbl)  [unwired: 2 in]
        n115 = call <vilib>:"compatOverwrite.vi"("overwrite (F)"=TRUE) -> ("overwrite?"=w363:T7)
        n116 = Bundle By Name(cluster=w391, "Drain Start"=w395, "Drain Stop"=w394, "Drain Step"=w393, "Drain Compliance"=w411, "Range mode"=w373, "Range"=w372) -> (w377:T4)
        n117 = call "4155C Transfer-FPP.vi"("VISA resource name in"=w379, "Gate"=w376, "Drain"=w377, "Timings"=w409, "error in (no error)"=w380, "sweep mode"=w401, "Panel Controls"=w426) -> ("VG"=w417:dbl[], "Outparams"=w371:T8, "VISA Resource Name out"=w407:refnum<visa-resource-name>, "Vprobe2"=w367:dbl[], "ID"=w366:dbl[], "IG"=w365:dbl[], "Vprobe1"=w364:dbl[], "error out"=w408:errorcluster)  [unwired: 13 in]
        n118 = Unbundle By Name(w371) -> ("V2 Step"=w370:dbl, "V2 Start"=w369:dbl, "Number of points"=w368:i32)
        n119 = Open/Create/Replace File(file path (use dialog)=w412, error in=w408, operation (0:open)=w363) -> (refnum out=w423:refnum<file>, error out=w424:errorcluster)  [unwired: 3 in, 1 out]
        n120 = call "4155C Make Big 2d array FPP.vi"("1D Var1"=w417, "1d ID"=w366, "1d Vp2"=w367, "1d IG"=w365, "1d Vp1"=w364, "VAR2 START"=w369, "Number of VAR2 steps"=w368, "VAR2 STEP"=w370, "VAR1 Name"="Vg", "Decimal places in header"=i8 1, "VAR2 Name"="Vd") -> ("Header array"=w419:string[], "Data array"=w420:dbl[][])  [unwired: 15 in]
        n121 = call "4155C Write array to file.vi"("Byte Stream File Refnum"=w423, "Header"=w419, "Data Array"=w420, "error in (no error)"=w424) -> ("dup refnum"=w421:refnum<file>, "error out"=w422:errorcluster)  [unwired: 1 in]
        n122 = Close File(refnum=w421, error in=w422) -> (error out=w406:errorcluster)  [unwired: 1 out]
      }
      frame "output" {
        n123 = Number To Decimal String(number=w431) -> (decimal integer string=w482:string)  [unwired: 1 in]
        n124 = Bundle By Name(cluster=w458, "Emergency Stop"=w489) -> (w499:T6)
        n125 = Delete From Array(array=w473, index=0 ("Index")) -> (deleted portion=w471:string, array with subset deleted=w470:string[])  [unwired: 1 in]
        n126 = Concatenate Strings(w481, "-output-" ("Substring"), w482, w430, ".txt" ("Substring")) -> (w484:string)
        n127 = VISA Write(VISA resource name=w449, write buffer=":PAGE:CHAN:MODE SWE;" ("write buffer (\"\")"), error in (no error)=w446) -> (VISA resource name out=w448:refnum<visa-resource-name>, error out=w447:errorcluster)  [unwired: 1 out]
        n128 = case shown="\"d\", Default" w471 {
          tunnel: [w500 w501] -> w469
          frame "s" {
            w500 = u16 0 items=["Single", "Double"] ("sweep mode")
          }
          frame "d", Default {
            w501 = u16 1 items=["Single", "Double"] ("sweep mode")
          }
        }
        n129 = Fract/Exp String To Number(string=w470) -> (number=w452:dbl[])  [unwired: 3 in, 1 out]
        n130 = String To Path(string=w484) -> (path=w480:path)
        n131 = Index Array(array=w452, index #1=0 ("Index")) -> (element #1=w468:dbl, element #2=w467:dbl, element #3=w466:dbl)  [unwired: 2 in]
        n132 = Delete From Array(array=w452, length=3 ("Length"), index=0 ("Index")) -> (array with subset deleted=w451:dbl[])  [unwired: 1 out]
        n133 = Bundle By Name(cluster=w460, "Gate Start"=w468, "Gate Stop"=w467, "Gate Step (linear only)"=w466, "Gate Compliance"=w478, "Range mode"=w444, "Range"=w443) -> (w498:T3)
        n134 = Index Array(array=w451, index #1=0 ("Index")) -> (element #1=w463:dbl, element #2=w462:dbl, element #3=w461:dbl)  [unwired: 2 in]
        n135 = call <vilib>:"compatOverwrite.vi"("overwrite (F)"=TRUE) -> ("overwrite?"=w435:T7)
        n136 = Bundle By Name(cluster=w459, "Drain Start"=w463, "Drain Stop"=w462, "Drain Step"=w461, "Drain Compliance"=w479, "Range mode"=w442, "Range"=w445) -> (w497:T4)
        n137 = call "4155C Output.vi"("VISA resource name in"=w448, "Gate"=w498, "Drain"=w497, "Timings"=w477, "error in (no error)"=w447, "SMU4"=w437, "sweep mode"=w469, "Panel controls"=w499) -> ("VD"=w485:dbl[], "Outparams"=w440:T8, "VISA Resource Name out"=w475:refnum<visa-resource-name>, "IS"=w488:dbl[], "ID"=w487:dbl[], "IG"=w486:dbl[], "error out"=w476:errorcluster, "SMU4"=w436:dbl[])  [unwired: 12 in]
        n138 = Unbundle By Name(w440) -> ("V2 Step"=w441:dbl, "V2 Start"=w439:dbl, "Number of points"=w438:i32)
        n139 = Open/Create/Replace File(file path (use dialog)=w480, error in=w476, operation (0:open)=w435) -> (refnum out=w494:refnum<file>, error out=w495:errorcluster)  [unwired: 3 in, 1 out]
        n140 = call "4155C Make Big 2d array.vi"("1D Var1"=w485, "1d IS"=w488, "1d ID"=w487, "1d IG"=w486, "1d SMU4"=w436, "SMU4"=w437, "VAR2 START"=w439, "Number of VAR2 steps"=w438, "VAR2 STEP"=w441, "VAR1 Name"="Vd", "Decimal places in header"=i8 1, "VAR2 Name"="Vg") -> ("Header array"=w490:string[], "Data array"=w491:dbl[][])  [unwired: 14 in]
        n141 = call "4155C Write array to file.vi"("Byte Stream File Refnum"=w494, "Header"=w490, "Data Array"=w491, "error in (no error)"=w495) -> ("dup refnum"=w492:refnum<file>, "error out"=w493:errorcluster)  [unwired: 1 in]
        n142 = Close File(refnum=w492, error in=w493) -> (error out=w474:errorcluster)  [unwired: 1 out]
      }
      frame "output-fpp" {
        n143 = Number To Decimal String(number=w504) -> (decimal integer string=w558:string)  [unwired: 1 in]
        n144 = Bundle By Name(cluster=w534, "Emergency Stop"=w561) -> (w571:T6)
        n145 = Delete From Array(array=w549, index=0 ("Index")) -> (deleted portion=w547:string, array with subset deleted=w546:string[])  [unwired: 1 in]
        n146 = VISA Write(VISA resource name=w525, write buffer=":PAGE:CHAN:MODE SWE;" ("write buffer (\"\")"), error in (no error)=w522) -> (VISA resource name out=w524:refnum<visa-resource-name>, error out=w523:errorcluster)  [unwired: 1 out]
        n147 = Concatenate Strings(w557, "-outputfpp-" ("Substring"), w558, w503, ".txt" ("Substring")) -> (w560:string)
        n148 = case shown="\"d\", Default" w547 {
          tunnel: [w572 w573] -> w545
          frame "s" {
            w572 = u16 0 items=["Single", "Double"] ("sweep mode")
          }
          frame "d", Default {
            w573 = u16 1 items=["Single", "Double"] ("sweep mode")
          }
        }
        n149 = Fract/Exp String To Number(string=w546) -> (number=w528:dbl[])  [unwired: 3 in, 1 out]
        n150 = String To Path(string=w560) -> (path=w556:path)
        n151 = Index Array(array=w528, index #1=0 ("Index")) -> (element #1=w544:dbl, element #2=w543:dbl, element #3=w542:dbl)  [unwired: 2 in]
        n152 = Delete From Array(array=w528, length=3 ("Length"), index=0 ("Index")) -> (array with subset deleted=w527:dbl[])  [unwired: 1 out]
        n153 = Bundle By Name(cluster=w536, "Gate Start"=w544, "Gate Stop"=w543, "Gate Step (linear only)"=w542, "Gate Compliance"=w554, "Range mode"=w520, "Range"=w519) -> (w570:T3)
        n154 = Index Array(array=w527, index #1=0 ("Index")) -> (element #1=w539:dbl, element #2=w538:dbl, element #3=w537:dbl)  [unwired: 2 in]
        n155 = call <vilib>:"compatOverwrite.vi"("overwrite (F)"=TRUE) -> ("overwrite?"=w508:T7)
        n156 = Bundle By Name(cluster=w535, "Drain Start"=w539, "Drain Stop"=w538, "Drain Step"=w537, "Drain Compliance"=w555, "Range mode"=w518, "Range"=w521) -> (w569:T4)
        n157 = call "4155C Output-FPP.vi"("VISA resource name in"=w524, "Gate"=w570, "Drain"=w569, "Timings"=w553, "error in (no error)"=w523, "sweep mode"=w545, "Panel controls"=w571) -> ("VD"=w513:dbl[], "Outparams"=w516:T8, "VISA Resource Name out"=w551:refnum<visa-resource-name>, "Vprobe2"=w512:dbl[], "ID"=w511:dbl[], "IG"=w510:dbl[], "Vprobe1"=w509:dbl[], "error out"=w552:errorcluster)  [unwired: 13 in]
        n158 = Unbundle By Name(w516) -> ("V2 Step"=w517:dbl, "V2 Start"=w515:dbl, "Number of points"=w514:i32)
        n159 = Open/Create/Replace File(file path (use dialog)=w556, error in=w552, operation (0:open)=w508) -> (refnum out=w566:refnum<file>, error out=w567:errorcluster)  [unwired: 3 in, 1 out]
        n160 = call "4155C Make Big 2d array FPP.vi"("1D Var1"=w513, "1d ID"=w511, "1d Vp2"=w512, "1d IG"=w510, "1d Vp1"=w509, "VAR2 START"=w515, "Number of VAR2 steps"=w514, "VAR2 STEP"=w517, "VAR1 Name"="Vd", "Decimal places in header"=i8 1, "VAR2 Name"="Vg") -> ("Header array"=w562:string[], "Data array"=w563:dbl[][])  [unwired: 15 in]
        n161 = call "4155C Write array to file.vi"("Byte Stream File Refnum"=w566, "Header"=w562, "Data Array"=w563, "error in (no error)"=w567) -> ("dup refnum"=w564:refnum<file>, "error out"=w565:errorcluster)  [unwired: 1 in]
        n162 = Close File(refnum=w564, error in=w565) -> (error out=w550:errorcluster)  [unwired: 1 out]
      }
      frame "itime" {
        n163 = Delete From Array(array=w588, index=0 ("Index")) -> (deleted portion=w589:string)  [unwired: 1 in, 1 out]
        n164 = case shown="\"l\"" w589 {
          tunnel: w587 -> [w593 w595 w598]
          tunnel: [w592 w594 w597] -> w580
          frame "s" {
            w591 = u32 0 items=["short  ", "medium  ", "long  "] ("integration time 2")
            n165 = Bundle By Name(cluster=w593, "integration time"=w591) -> (w592:T5)
          }
          frame "m", Default {
            w596 = u32 1 items=["short  ", "medium  ", "long  "] ("integration time 2")
            n166 = Bundle By Name(cluster=w595, "integration time"=w596) -> (w594:T5)
          }
          frame "l" {
            w599 = u32 2 items=["short  ", "medium  ", "long  "] ("integration time 2")
            n167 = Bundle By Name(cluster=w598, "integration time"=w599) -> (w597:T5)
          }
        }
      }
      frame "pulsed" {
        n168 = Delete From Array(array=w615, index=0 ("Index")) -> (deleted portion=w616:string, array with subset deleted=w603:string[])  [unwired: 1 in]
        n169 = case shown="\"on\", Default" w616 {
          tunnel: w614 -> [w626 w629]
          tunnel: [w625 w628] -> w607
          tunnel: w603 -> [w623 _]
          frame "on", Default {
            w624 = u16 1 items=["Continuous", "Pulsed"] ("sweep method")
            n170 = Fract/Exp String To Number(string=w623) -> (number=w621:dbl[])  [unwired: 3 in, 1 out]
            n171 = Index Array(array=w621, index #1=0 ("Index")) -> (element #1=w620:dbl, element #2=w619:dbl, element #3=w618:dbl)  [unwired: 2 in]
            n172 = Bundle By Name(cluster=w626, "sweep method"=w624, "Pulse period"=w620, "Base voltage"=w619, "Pulse width"=w618) -> (w625:T5)
          }
          frame "off" {
            w627 = u16 0 items=["Continuous", "Pulsed"] ("sweep method")
            n173 = Bundle By Name(cluster=w629, "sweep method"=w627) -> (w628:T5)
          }
        }
      }
      frame "gaterangemode" {
        n174 = Delete From Array(array=w643, index=0 ("Index")) -> (deleted portion=w644:string)  [unwired: 1 in, 1 out]
        n175 = case shown="\"f\"" w644 {
          tunnel: [w646 w647 w648] -> w633
          frame "a", Default {
            w646 = u16 0 items=["Auto", "Limited", "Fixed"] ("Gate Range\nmode 2")
          }
          frame "f" {
            w647 = u16 2 items=["Auto", "Limited", "Fixed"] ("Gate Range\nmode 2")
          }
          frame "l" {
            w648 = u16 1 items=["Auto", "Limited", "Fixed"] ("Gate Range\nmode 2")
          }
        }
      }
      frame "gaterange" {
        (unwired) u8 11 items=["10fA  ", "100fA  ", "1nA  ", "10nA", "100nA", "1uA", "10uA", "100uA", "1mA", "10mA", "100mA", "1A"] ("Gate Range 2")
        n176 = Delete From Array(array=w669, index=0 ("Index")) -> (deleted portion=w659:string)  [unwired: 1 in, 1 out]
        n177 = Scan Value(string=w659, format string="") -> (value=w657:dbl)  [unwired: 1 in, 1 out]
        n178 = Logarithm Base 10(1:w657) -> (0:w656:dbl)
        n179 = Round To Nearest(number=w656) -> (nearest integer value=w655:dbl)
        n180 = Add(x=w655, y=11.0) -> (x+y=w653:dbl)
        n181 = To Unsigned Byte Integer(number=w653) -> (unsigned 8bit integer=w652:u8)
      }
      frame "drainrange" {
        (unwired) u8 11 items=["10fA  ", "100fA  ", "1nA  ", "10nA", "100nA", "1uA", "10uA", "100uA", "1mA", "10mA", "100mA", "1A"] ("Gate Range 2")
        n182 = Delete From Array(array=w691, index=0 ("Index")) -> (deleted portion=w682:string)  [unwired: 1 in, 1 out]
        n183 = Scan Value(string=w682, format string="") -> (value=w680:dbl)  [unwired: 1 in, 1 out]
        n184 = Logarithm Base 10(1:w680) -> (0:w679:dbl)
        n185 = Round To Nearest(number=w679) -> (nearest integer value=w678:dbl)
        n186 = Add(x=w678, y=11.0) -> (x+y=w676:dbl)
        n187 = To Unsigned Byte Integer(number=w676) -> (unsigned 8bit integer=w675:u8)
      }
      frame "drainrangemode" {
        n188 = Delete From Array(array=w706, index=0 ("Index")) -> (deleted portion=w707:string)  [unwired: 1 in, 1 out]
        n189 = case shown="\"f\"" w707 {
          tunnel: [w709 w710 w711] -> w696
          frame "a", Default {
            w709 = u16 0 items=["Auto", "Limited", "Fixed"] ("Gate Range\nmode 2")
          }
          frame "f" {
            w710 = u16 2 items=["Auto", "Limited", "Fixed"] ("Gate Range\nmode 2")
          }
          frame "l" {
            w711 = u16 1 items=["Auto", "Limited", "Fixed"] ("Gate Range\nmode 2")
          }
        }
      }
      frame "Error", Default {
      }
      frame "logfile" {
        n190 = Number To Decimal String(number=w728) -> (decimal integer string=w763:string)  [unwired: 1 in]
        n191 = Concatenate Strings(w762, "logfile" ("Substring"), w763, w726, ".txt" ("Substring")) -> (w760:string)
        n192 = String To Path(string=w760) -> (path=w733:path)
        n193 = Unbundle(w759) -> ("integration time"=w758:u32, "Short/Long integration time"=w757:dbl, "hold time (sec)"=w756:dbl, "delay time (sec)"=w755:dbl, "Step Time (0 disables)"=w754:dbl, "sweep method"=w753:u16, "Pulse period"=w752:dbl, "Base voltage"=w751:dbl, "Pulse width"=w750:dbl)
        n194 = Build Array(w758, w757, w756, w755, w754, w753, w752, w751, w750, w744, w745, w746, w747, w748, w749) -> (w737:dbl[])
        n195 = Insert Into Array(array=dbl[][] [] ("Input Array"), new element=w737) -> (w736:dbl[][])  [unwired: 2 in]
        n196 = call <vilib>:"compatOverwrite.vi"("overwrite (F)"=TRUE) -> ("overwrite?"=w731:T7)
        n197 = Open/Create/Replace File(file path (use dialog)=w733, error in=w735, operation (0:open)=w731) -> (refnum out=w741:refnum<file>, error out=w740:errorcluster)  [unwired: 3 in, 1 out]
        n198 = call "4155C Write array to file.vi"("Byte Stream File Refnum"=w741, "Header"=string[] ["Int Time", "Short/Long Itime", "Hold time", "Delay time", "Step time", "Sweep method", "Pulse period", "Base Voltage", "Pulse width", "Drain compliance", "Gate compliance", "Gate range mode", "Gate range", "S/D range mode", "S/D range"], "Data Array"=w736, "error in (no error)"=w740) -> ("dup refnum"=w743:refnum<file>, "error out"=w742:errorcluster)  [unwired: 1 in]
        n199 = Close File(refnum=w743, error in=w742) -> (error out=w734:errorcluster)  [unwired: 1 out]
      }
      frame "sample" {
        n200 = Number To Decimal String(number=w768) -> (decimal integer string=w816:string)  [unwired: 1 in]
        n201 = Fract/Exp String To Number(string=w813) -> (number=w774:dbl[])  [unwired: 3 in, 1 out]
        n202 = Concatenate Strings(w791, "-sample-" ("Substring"), w816, w766, ".txt" ("Substring")) -> (w814:string)
        n203 = String To Path(string=w814) -> (path=w795:path)
        n204 = Index Array(array=w774, index=0 ("Index")) -> (element=w811:dbl)
        n205 = Index Array(array=w774, index=2 ("Index")) -> (element=w807:dbl)
        n206 = Index Array(array=w774, index=3 ("Index")) -> (element=w776:dbl)
        n207 = Index Array(array=w774, index=4 ("Index")) -> (element=w773:dbl)
        n208 = call "4155C Config Sampling Measurements.vi"("Sampling interval"=w773, "Sample time"=w776, "Display on/off"=TRUE, "Timings"=w782, "Num Points"=w807, "error in (no error)"=w818, "Drain Compliance"=w817, "Gate Compliance"=w792, "VISA session"=w819) -> ("error out"=w820:errorcluster, "dup VISA resource name"=w821:refnum<visa-resource-name>)  [unwired: 1 in]
        n209 = Index Array(array=w774, index=1 ("Index")) -> (element=w808:dbl)
        n210 = call "4155C Take Sample.vi"("Emergency Stop"=w788, "error in (no error)"=w820, "Vd"=w808, "Vg"=w811, "VISA resource name in"=w821) -> ("error out"=w786:errorcluster, "Id"=w823:dbl[], "Ig"=w797:dbl[], "VISA Resource Name out"=w784:refnum<visa-resource-name>, "Is"=w822:dbl[], "Time"=w801:dbl[])  [unwired: 1 in]
        n211 = Insert Into Array(array=dbl[][] [] ("Input Array"), new element=w801) -> (w800:dbl[][])  [unwired: 2 in]
        n212 = Insert Into Array(array=w800, new element=w797) -> (w799:dbl[][])  [unwired: 2 in]
        n213 = Insert Into Array(array=w799, new element=w823) -> (w798:dbl[][])  [unwired: 2 in]
        n214 = VISA Write(VISA resource name=w784, write buffer=":DISP ON" ("write buffer (\"\")"), error in (no error)=w786) -> (VISA resource name out=w783:refnum<visa-resource-name>, error out=w785:errorcluster)  [unwired: 1 out]
        n215 = Insert Into Array(array=w798, new element=w822) -> (w790:dbl[][])  [unwired: 2 in]
        n216 = Transpose 2D Array(2D array=w790) -> (transposed array=w789:dbl[][])
        n217 = call <vilib>:"compatOverwrite.vi"("overwrite (F)"=TRUE) -> ("overwrite?"=w771:T7)
        n218 = Open/Create/Replace File(file path (use dialog)=w795, error in=w785, operation (0:open)=w771) -> (refnum out=w804:refnum<file>, error out=w803:errorcluster)  [unwired: 3 in, 1 out]
        n219 = call "4155C Write array to file.vi"("Byte Stream File Refnum"=w804, "Header"=string[] ["Time /s", "Ig /A", "Id /A", "Is /A"], "Data Array"=w789, "error in (no error)"=w803) -> ("dup refnum"=w806:refnum<file>, "error out"=w805:errorcluster)  [unwired: 1 in]
        n220 = Close File(refnum=w806, error in=w805) -> (error out=w793:errorcluster)  [unwired: 1 out]
      }
      frame "samplei" {
        n221 = Number To Decimal String(number=w826) -> (decimal integer string=w878:string)  [unwired: 1 in]
        n222 = Fract/Exp String To Number(string=w875) -> (number=w842:dbl[])  [unwired: 3 in, 1 out]
        n223 = Concatenate Strings(w857, "-samplei-" ("Substring"), w878, w825, ".txt" ("Substring")) -> (w876:string)
        n224 = String To Path(string=w876) -> (path=w860:path)
        n225 = Index Array(array=w842, index=4 ("Index")) -> (element=w836:dbl)
        n226 = Index Array(array=w842, index=3 ("Index")) -> (element=w837:dbl)
        n227 = Index Array(array=w842, index=1 ("Index")) -> (element=w839:dbl)
        n228 = Index Array(array=w842, index=0 ("Index")) -> (element=w840:dbl)
        n229 = Index Array(array=w842, index=2 ("Index")) -> (element=w838:dbl)
        n230 = call "4155C Config SamplingI Measurements.vi"("Sample time"=w838, "Display on/off"=TRUE, "Timings"=w849, "Num Points"=w839, "error in (no error)"=w880, "Sampling interval"=w837, "VISA session"=w881) -> ("error out"=w882:errorcluster, "dup VISA resource name"=w883:refnum<visa-resource-name>)  [unwired: 3 in]
        n231 = call "4155C Take SampleI.vi"("Emergency Stop"=w854, "error in (no error)"=w882, "Idg 2"=w840, "Vdg compliance 2"=w836, "VISA resource name in"=w883) -> ("error out"=w852:errorcluster, "Idg"=w885:dbl[], "Vdg"=w862:dbl[], "VISA Resource Name out"=w850:refnum<visa-resource-name>, "Is"=w884:dbl[], "Time"=w866:dbl[])  [unwired: 1 in]
        n232 = Insert Into Array(array=dbl[][] [] ("Input Array"), new element=w866) -> (w865:dbl[][])  [unwired: 2 in]
        n233 = Insert Into Array(array=w865, new element=w862) -> (w864:dbl[][])  [unwired: 2 in]
        n234 = Insert Into Array(array=w864, new element=w885) -> (w863:dbl[][])  [unwired: 2 in]
        n235 = VISA Write(VISA resource name=w850, write buffer=":DISP ON" ("write buffer (\"\")"), error in (no error)=w852) -> (VISA resource name out=w835:refnum<visa-resource-name>, error out=w851:errorcluster)  [unwired: 1 out]
        n236 = Insert Into Array(array=w863, new element=w884) -> (w856:dbl[][])  [unwired: 2 in]
        n237 = Transpose 2D Array(2D array=w856) -> (transposed array=w855:dbl[][])
        n238 = call <vilib>:"compatOverwrite.vi"("overwrite (F)"=TRUE) -> ("overwrite?"=w830:T7)
        n239 = Open/Create/Replace File(file path (use dialog)=w860, error in=w851, operation (0:open)=w830) -> (refnum out=w869:refnum<file>, error out=w868:errorcluster)  [unwired: 3 in, 1 out]
        n240 = call "4155C Write array to file.vi"("Byte Stream File Refnum"=w869, "Header"=string[] ["Time /s", "Vdg /V", "Idg /A", "Is /A"], "Data Array"=w855, "error in (no error)"=w868) -> ("dup refnum"=w871:refnum<file>, "error out"=w870:errorcluster)  [unwired: 1 in]
        n241 = Close File(refnum=w871, error in=w870) -> (error out=w833:errorcluster)  [unwired: 1 out]
        n242 = VISA Write(VISA resource name=w835, write buffer=";:PAGE:SCON:STAN OFF;:PAGE:CHAN:VSU2:DIS;" ("write buffer (\"\")"), error in (no error)=w833) -> (VISA resource name out=w831:refnum<visa-resource-name>, error out=w832:errorcluster)  [unwired: 1 out]
      }
      frame "#" {
        n243 = VISA Write(VISA resource name=w893, write buffer=":DISP ON" ("write buffer (\"\")"), error in (no error)=w892) -> (VISA resource name out=w891:refnum<visa-resource-name>, error out=w890:errorcluster)  [unwired: 1 out]
      }
      frame "stressV" {
        n244 = Number To Decimal String(number=w904) -> (decimal integer string=w945:string)  [unwired: 1 in]
        n245 = Fract/Exp String To Number(string=w942) -> (number=w915:dbl[])  [unwired: 3 in, 1 out]
        n246 = Concatenate Strings(w929, "-stressV-" ("Substring"), w945, w903, ".txt" ("Substring")) -> (w943:string)
        n247 = String To Path(string=w943) -> (path=w933:path)
        n248 = Index Array(array=w915, index=3 ("Index")) -> (element=w912:dbl)
        n249 = Index Array(array=w915, index=1 ("Index")) -> (element=w910:dbl)
        n250 = Index Array(array=w915, index=0 ("Index")) -> (element=w909:dbl)
        n251 = Index Array(array=w915, index=4 ("Index")) -> (element=w914:dbl)
        n252 = Index Array(array=w915, index=2 ("Index")) -> (element=w911:dbl)
        n253 = call "4155C Config V Stress.vi"("VISA session"=w948, "ID compliance"=w912, "VD"=w910, "VG"=w909, "IG compliance"=w911, "error in (no error)"=w947, "Display on/off"=TRUE) -> ("dup VISA resource name"=w950:refnum<visa-resource-name>, "error out"=w949:errorcluster)
        n254 = call "4155C Apply Stress.vi"("error in (no error)"=w949, "Duration"=w914, "Emergency Stop"=w928, "VISA resource name in"=w950) -> ("error out"=w926:errorcluster, "VISA Resource Name out"=w924:refnum<visa-resource-name>)
        n255 = VISA Write(VISA resource name=w924, write buffer=":DISP ON" ("write buffer (\"\")"), error in (no error)=w926) -> (VISA resource name out=w923:refnum<visa-resource-name>, error out=w925:errorcluster)  [unwired: 1 out]
        n256 = call <vilib>:"compatOverwrite.vi"("overwrite (F)"=TRUE) -> ("overwrite?"=w908:T7)
        n257 = Open/Create/Replace File(file path (use dialog)=w933, error in=w925, operation (0:open)=w908) -> (refnum out=w936:refnum<file>, error out=w935:errorcluster)  [unwired: 3 in, 1 out]
        n258 = call "4155C Write array to file.vi"("Byte Stream File Refnum"=w936, "Header"=string[] ["V stress completed successfully", ""], "error in (no error)"=w935) -> ("dup refnum"=w938:refnum<file>, "error out"=w937:errorcluster)  [unwired: 2 in]
        n259 = Close File(refnum=w938, error in=w937) -> (error out=w931:errorcluster)  [unwired: 1 out]
      }
      frame "stressI" {
        n260 = Number To Decimal String(number=w953) -> (decimal integer string=w990:string)  [unwired: 1 in]
        n261 = Fract/Exp String To Number(string=w987) -> (number=w962:dbl[])  [unwired: 3 in, 1 out]
        n262 = Concatenate Strings(w974, "-stressI-" ("Substring"), w990, w952, ".txt" ("Substring")) -> (w988:string)
        n263 = String To Path(string=w988) -> (path=w978:path)
        n264 = Index Array(array=w962, index=1 ("Index")) -> (element=w958:dbl)
        n265 = Index Array(array=w962, index=0 ("Index")) -> (element=w959:dbl)
        n266 = call "4155C Config I Stress.vi"("VISA session"=w993, "IDG"=w959, "VDG compliance"=w958, "error in (no error)"=w992, "Display on/off"=TRUE) -> ("dup VISA resource name"=w995:refnum<visa-resource-name>, "error out"=w994:errorcluster)
        n267 = Index Array(array=w962, index=2 ("Index")) -> (element=w960:dbl)
        n268 = call "4155C Apply Stress.vi"("error in (no error)"=w994, "Duration"=w960, "Emergency Stop"=w973, "VISA resource name in"=w995) -> ("error out"=w971:errorcluster, "VISA Resource Name out"=w969:refnum<visa-resource-name>)
        n269 = VISA Write(VISA resource name=w969, write buffer=":DISP ON" ("write buffer (\"\")"), error in (no error)=w971) -> (VISA resource name out=w968:refnum<visa-resource-name>, error out=w970:errorcluster)  [unwired: 1 out]
        n270 = call <vilib>:"compatOverwrite.vi"("overwrite (F)"=TRUE) -> ("overwrite?"=w957:T7)
        n271 = Open/Create/Replace File(file path (use dialog)=w978, error in=w970, operation (0:open)=w957) -> (refnum out=w981:refnum<file>, error out=w980:errorcluster)  [unwired: 3 in, 1 out]
        n272 = call "4155C Write array to file.vi"("Byte Stream File Refnum"=w981, "Header"=string[] ["I stress completed successfully", ""], "error in (no error)"=w980) -> ("dup refnum"=w983:refnum<file>, "error out"=w982:errorcluster)  [unwired: 2 in]
        n273 = Close File(refnum=w983, error in=w982) -> (error out=w976:errorcluster)  [unwired: 1 out]
      }
      frame "vsu2pulse" {
        n274 = Number To Decimal String(number=w998) -> (decimal integer string=w1033:string)  [unwired: 1 in]
        n275 = Fract/Exp String To Number(string=w1030) -> (number=w1006:dbl[])  [unwired: 3 in, 1 out]
        n276 = Concatenate Strings(w1018, "-vsu2-" ("Substring"), w1033, w997, ".txt" ("Substring")) -> (w1031:string)
        n277 = String To Path(string=w1031) -> (path=w1022:path)
        n278 = Index Array(array=w1006, index=1 ("Index")) -> (element=w1005:dbl)
        n279 = Index Array(array=w1006, index=0 ("Index")) -> (element=w1003:dbl)
        n280 = call "4155C Config VSU2 Stress.vi"("error in (no error)"=w1035, "VSU2"=w1003, "Display on/off"=TRUE, "VISA session"=w1036) -> ("error out"=w1037:errorcluster, "dup VISA resource name"=w1038:refnum<visa-resource-name>)
        n281 = call "4155C Apply Stress.vi"("error in (no error)"=w1037, "Duration"=w1005, "Emergency Stop"=w1017, "VISA resource name in"=w1038) -> ("error out"=w1015:errorcluster, "VISA Resource Name out"=w1013:refnum<visa-resource-name>)
        n282 = VISA Write(VISA resource name=w1013, write buffer=":DISP ON" ("write buffer (\"\")"), error in (no error)=w1015) -> (VISA resource name out=w1012:refnum<visa-resource-name>, error out=w1014:errorcluster)  [unwired: 1 out]
        n283 = call <vilib>:"compatOverwrite.vi"("overwrite (F)"=TRUE) -> ("overwrite?"=w1002:T7)
        n284 = Open/Create/Replace File(file path (use dialog)=w1022, error in=w1014, operation (0:open)=w1002) -> (refnum out=w1025:refnum<file>, error out=w1024:errorcluster)  [unwired: 3 in, 1 out]
        n285 = call "4155C Write array to file.vi"("Byte Stream File Refnum"=w1025, "Header"=string[] ["VSU2 pulse completed successfully", ""], "error in (no error)"=w1024) -> ("dup refnum"=w1027:refnum<file>, "error out"=w1026:errorcluster)  [unwired: 2 in]
        n286 = Close File(refnum=w1027, error in=w1026) -> (error out=w1020:errorcluster)  [unwired: 1 out]
      }
      frame "sample-fpp" {
        w1052 = string[] ["Time /s", "Id VgVd /A", "Ig VgVd /A", "Vp1 VgVd /V", "Vp2 VgVd /V"] ("Header")
        w1056 = "%d" ("format string")
        n287 = Number To Decimal String(number=w1041) -> (decimal integer string=w1104:string)  [unwired: 1 in]
        n288 = Fract/Exp String To Number(string=w1101) -> (number=w1089:dbl[])  [unwired: 3 in, 1 out]
        n289 = Concatenate Strings(w1095, "-samplefpp-" ("Substring"), w1104, w1040, ".txt" ("Substring")) -> (w1102:string)
        n290 = String To Path(string=w1102) -> (path=w1064:path)
        n291 = Index Array(array=w1089, index=0 ("Index")) -> (element=w1050:dbl)
        n292 = Index Array(array=w1089, index=1 ("Index")) -> (element=w1049:dbl)
        n293 = Index Array(array=w1089, index=2 ("Index")) -> (element=w1097:dbl)
        n294 = Index Array(array=w1089, index=3 ("Index")) -> (element=w1087:dbl)
        n295 = call "4155C Config Sampling Measurements FPP.vi"("VISA session"=w1107, "Num Points"=w1097, "Vg"=w1050, "Display on/off"=TRUE, "Gate Compliance"=w1096, "Drain Compliance"=w1105, "Standby"="Standby", "error in (no error)"=w1106, "Timings"=w1094, "Vd"=w1049, "Sample time"=w1087) -> ("dup VISA resource name"=w1066:refnum<visa-resource-name>, "error out"=w1065:errorcluster)  [unwired: 3 in]
        n296 = Number To Decimal String(number=w1050) -> (decimal integer string=w1076:string)  [unwired: 1 in]
        n297 = call "4155C Take Sample FPP.vi"("VISA resource name in"=w1066, "error in (no error)"=w1065, "Emergency Stop"=w1067) -> ("Time"=w1071:dbl[], "Vp1"=w1081:dbl[], "VISA Resource Name out"=w1047:refnum<visa-resource-name>, "Ig"=w1069:dbl[], "Id"=w1070:dbl[], "Vp2"=w1079:dbl[], "error out"=w1068:errorcluster)  [unwired: 10 in]
        n298 = Insert Into Array(array=dbl[][] [] ("Input Array"), new element=w1071) -> (w1085:dbl[][])  [unwired: 2 in]
        n299 = Number To Decimal String(number=w1049) -> (decimal integer string=w1074:string)  [unwired: 1 in]
        n300 = Insert Into Array(array=w1085, new element=w1070) -> (w1084:dbl[][])  [unwired: 2 in]
        n301 = Concatenate Strings("(Vg = " ("Substring"), w1076, "V, Vd = " ("Substring"), w1074, "V)" ("Substring")) -> (w1072:string)
        n302 = Insert Into Array(array=w1084, new element=w1069) -> (w1083:dbl[][])  [unwired: 2 in]
        n303 = Insert Into Array(array=w1083, new element=w1081) -> (w1080:dbl[][])  [unwired: 2 in]
        n304 = Insert Into Array(array=w1080, new element=w1079) -> (w1048:dbl[][])  [unwired: 2 in]
        n305 = call <vilib>:"compatOverwrite.vi"("overwrite (F)"=TRUE) -> ("overwrite?"=w1045:T7)
        n306 = Open/Create/Replace File(file path (use dialog)=w1064, error in=w1068, operation (0:open)=w1045) -> (refnum out=w1061:refnum<file>, error out=w1062:errorcluster)  [unwired: 3 in, 1 out]
        n307 = Array To Spreadsheet String(array=w1052, 3:w1056) -> (spreadsheet string=w1058:string)  [unwired: 1 in]
        n308 = Transpose 2D Array(2D array=w1048) -> (transposed array=w1078:dbl[][])
        n309 = Search and Replace String(replace all?=TRUE ("replace all? (F)"), input string=w1058, search string="VgVd", replace string=w1072) -> (result string=w1054:string)  [unwired: 4 in, 3 out]
        n310 = Spreadsheet String To Array(format string=w1056, spreadsheet string=w1054, array type (2D Dbl)=w1052) -> (array=w1053:string[])  [unwired: 1 in]
        n311 = call "4155C Write array to file.vi"("Byte Stream File Refnum"=w1061, "Header"=w1053, "Data Array"=w1078, "error in (no error)"=w1062) -> ("dup refnum"=w1059:refnum<file>, "error out"=w1060:errorcluster)  [unwired: 1 in]
        n312 = Close File(refnum=w1059, error in=w1060) -> (error out=w1046:errorcluster)  [unwired: 1 out]
      }
      frame "resample-fpp" {
        w1123 = string[] ["Time /s", "Id VgVd /A", "Ig VgVd /A", "Vp1 VgVd /V", "Vp2 VgVd /V"] ("Header")
        w1127 = "%d" ("format string")
        n313 = Number To Decimal String(number=w1109) -> (decimal integer string=w1167:string)  [unwired: 1 in]
        n314 = Fract/Exp String To Number(string=w1164) -> (number=w1116:dbl[])  [unwired: 3 in, 1 out]
        n315 = Concatenate Strings(w1160, "-resamplefpp-" ("Substring"), w1167, w1110, ".txt" ("Substring")) -> (w1165:string)
        n316 = String To Path(string=w1165) -> (path=w1135:path)
        n317 = Index Array(array=w1116, index=0 ("Index")) -> (element=w1122:dbl)
        n318 = Index Array(array=w1116, index=1 ("Index")) -> (element=w1121:dbl)
        n319 = Number To Decimal String(number=w1122) -> (decimal integer string=w1145:string)  [unwired: 1 in]
        n320 = call "4155C Take Sample FPP.vi"("VISA resource name in"=w1118, "error in (no error)"=w1117, "Emergency Stop"=w1136) -> ("Time"=w1140:dbl[], "Vp1"=w1150:dbl[], "VISA Resource Name out"=w1120:refnum<visa-resource-name>, "Ig"=w1138:dbl[], "Id"=w1139:dbl[], "Vp2"=w1148:dbl[], "error out"=w1137:errorcluster)  [unwired: 10 in]
        n321 = Insert Into Array(array=dbl[][] [] ("Input Array"), new element=w1140) -> (w1154:dbl[][])  [unwired: 2 in]
        n322 = Number To Decimal String(number=w1121) -> (decimal integer string=w1143:string)  [unwired: 1 in]
        n323 = Insert Into Array(array=w1154, new element=w1139) -> (w1153:dbl[][])  [unwired: 2 in]
        n324 = Concatenate Strings("(Vg = " ("Substring"), w1145, "V, Vd = " ("Substring"), w1143, "V)" ("Substring")) -> (w1141:string)
        n325 = Insert Into Array(array=w1153, new element=w1138) -> (w1152:dbl[][])  [unwired: 2 in]
        n326 = Insert Into Array(array=w1152, new element=w1150) -> (w1149:dbl[][])  [unwired: 2 in]
        n327 = Insert Into Array(array=w1149, new element=w1148) -> (w1115:dbl[][])  [unwired: 2 in]
        n328 = call <vilib>:"compatOverwrite.vi"("overwrite (F)"=TRUE) -> ("overwrite?"=w1114:T7)
        n329 = Open/Create/Replace File(file path (use dialog)=w1135, error in=w1137, operation (0:open)=w1114) -> (refnum out=w1132:refnum<file>, error out=w1133:errorcluster)  [unwired: 3 in, 1 out]
        n330 = Array To Spreadsheet String(array=w1123, 3:w1127) -> (spreadsheet string=w1129:string)  [unwired: 1 in]
        n331 = Transpose 2D Array(2D array=w1115) -> (transposed array=w1147:dbl[][])
        n332 = Search and Replace String(replace all?=TRUE ("replace all? (F)"), input string=w1129, search string="VgVd", replace string=w1141) -> (result string=w1125:string)  [unwired: 4 in, 3 out]
        n333 = Spreadsheet String To Array(format string=w1127, spreadsheet string=w1125, array type (2D Dbl)=w1123) -> (array=w1124:string[])  [unwired: 1 in]
        n334 = call "4155C Write array to file.vi"("Byte Stream File Refnum"=w1132, "Header"=w1124, "Data Array"=w1147, "error in (no error)"=w1133) -> ("dup refnum"=w1130:refnum<file>, "error out"=w1131:errorcluster)  [unwired: 1 in]
        n335 = Close File(refnum=w1130, error in=w1131) -> (error out=w1119:errorcluster)  [unwired: 1 out]
      }
      frame "serial" {
        n336 = Index Array(array=w1172, index=0 ("Index")) -> (element=w1171:string)
        n337 = call "Serial write and read v0.4.vi"("Termination char\n(0xA = '\\n' = LF)\n(0xD = '\\r' = CR)"="Termination char\n(0xA = '\\n' = LF)\n(0xD = '\\r' = CR)", "Enable Termination\nChar (T)"="Enable Termination\nChar (T)", "parity"="parity", "stop bits"="stop bits", "string to write"=w1171, "flow control"="flow control", "byte count"="byte count", "Serial Settings:Serial End Mode for Reads"="Serial Settings:Serial End Mode for Reads", "Timeout (ms)"="Timeout (ms)", "error in (no error)"=w1177, "VISA resource name"="VISA resource name", "baud rate"="baud rate", "data bits"="data bits") -> ("read string"=→"Serial port output":string, "error out"=w1176:errorcluster)  [unwired: 1 in]
      }
    }
    n338 = Build Array("Time /s" ("element"), "Id max /A" ("VAR2 Name"), "Id min /A" ("VAR2 Name")) -> (w63:string[])
    n339 = Build Array(w58, w57, w48) -> (w56:dbl[][])
    n340 = Transpose 2D Array(2D array=w56) -> (transposed array=w55:dbl[][])
    n341 = Concatenate Strings(w54, "-Ion-", ".txt" ("Suffix")) -> (w71:string)
    n342 = Array To Spreadsheet String(array=w63, 3:"" ("format string")) -> (spreadsheet string=w62:string)  [unwired: 1 in]
    n343 = Array To Spreadsheet String(array=w55, 3:"%e" ("format string")) -> (spreadsheet string=w61:string)  [unwired: 1 in]
    n344 = String To Path(string=w71) -> (path=w70:path)
    n345 = Build Array(w62, w61) -> (w60:string[])
    n346 = Write to Text File(file (use dialog)=w70, text=w60, error in=w51) -> (refnum out=w72:refnum<file>, error out=w59:errorcluster)  [unwired: 1 in, 1 out]
    n347 = Close File(refnum=w72, error in=w59) -> (error out=w50:errorcluster)  [unwired: 1 out]
    "Line running" <- w82
    "Total lines" <- w81
  }
  "error out" <- w1
